vi "SIcamera_Manager- old.vi"() -> ()   [LabVIEW 2015]
uses:
  SI_Client_Subvis/Client Acquisition Mode Menu.ctl
  SI_Client_Subvis/Frame Mode 1.ctl
  SystemUtil/Command.ctl
  SI_Client_Subvis/CameraStates.ctl
  Log/LogItem.ctl
  GPS_Drivers/GPS_Driver_Global.vi
  TCS_Link/TCSLINK_global.vi
  Instance          36 24Saved   SIcamera_Manager .vi
  GUI/GSP_GUI_global.vi
  Apogee_Global.vi
panel:
  in  "CCD ROI Mode":u16(ring)=10 items=["Imaging, 1x1  "=0, "Imaging, 2x2"=1, "Imaging, 3x3"=2, "Spectroscopic, 1x1"=3, "Spectroscopic, 2x2"=4, "Spectroscopic, 3x3"=5, "MOS, 1x1"=11, "MOS, 2x2"=12, "MOS, 3x3"=13, "Slicer"=6, "Spectroscopic, ZZ Ceti"=14, "Slit Imaging/Alignment"=7, "MOS Imaging/Alignment"=10, "Set user-defined ROI..."=8, "Custom Mode"=9]
  in  "MOS":bool
  in  "Save As":u16(ring)=1 items=["U16 FITS", "I16 FITS", "I32 FITS", "SGL FITS", "U16 TIFF", "I16 TIFF", "I32 TIFF", "SGL TIFF"]
  in  "Port Readout":u16(ring)=2 items=["4-port", "Port A", "Port B", "Port C", "Port D"]
  in  "Lamp Cluster":T1
  out "Current File Name":string
  in  "Calculate Offset":bool
  in  "sy1":dbl
  in  "sx1":dbl
  in  "oy1":dbl
  in  "ox1":dbl
  in  "N/S Offset":dbl min=0.0 max=420.0 step=0.15 format="%03.2f"
  in  "N/S Offset Choice":u16(ring) items=["North", "South"]
  in  "E/W Offset Choice":u8(ring) items=["East", "West"]
  in  "E/W Offset":dbl min=0.0 max=420.0 step=0.15 format="%03.2f"
  in  "Offset Telescope":bool
  out "TCP/IP ID":refnum<k5>
  in  "Systems Status & Control":enum32{"Camera TCP/IP", "General"}(tab)
  in  "Reset TCP":bool
  in  "Get Camera Status":bool
  out "CCD Temp.":sgl
  out "Vacuum Pressure":sgl format="%#.4g"
  out "Connection Status":bool
  in  "Port":u16=2055
  in  "Server Address":string="Localhost"
  in  "Reset Wavelength Angles System":bool
  in  "Proposal #":string
  in  "Observer Name":string
  in  "Show Images?":bool
  out "CCD ROI":cluster{i32, i32, i32, i32, i32, i32}={0, 4096, 1, 0, 4096, 1}
  in  "CCD Readout Speed":u8(ring)=5 items=["50 kHz, ATTN 0", "50 kHz, ATTN 2", "50 kHz, ATTN 3", "100 kHz, ATTN 0", "100 kHz, ATTN 2", "100 kHz, ATTN 3", "200 kHz, ATTN 0", "200 kHz, ATTN 2", "400 kHz, ATTN 0"]
  out "Open Shutter During Image?":bool=TRUE
  out "Readout Time":dbl
  out "Image File Name":string="0001.image.fits"
  in  "Image #":i32=1 min=1 step=1 format="%04.0f"
  in  "Thumbnail Setting":enum16{"Check Entire CCD", "Check Star Focus"}(ring)
  in  "Take Thumbnail":bool
  out "Current Status":string
  in  "Save":bool
  in  "Frames":i32=1 min=1 step=1
  in  "Frame Mode":T2 items=["Single Frame Buffer", "Multiple Frame Buffer"]
  in  "Exp. Time (s)":dbl=1.0 min=0.5 step=1.0 format="%.1f"
  out "Packet\nError code":i32
  out "Function #":u16
  in  "# to Average":u32=2 caption="of"
  in  "RO Done":bool
  out "% Exposure":u16(slide) scale=0.0..100.0
  out "% Complete":u16(slide) caption="% Readout" scale=0.0..100.0
  out "Error out":errorcluster
  out "Acquiring":u32
  out "P Len":i32
  out "S Len":i32
  in  "Mode":u16(ring)=4 items=["Retrieve Image Buffer", "Acquire and transfer to client", "Acquire and hold in Server Image Buffer", "Acquire, transfer to client, and save to Server's disk", "Acquire, save to Server's disk, and hold in Server Image Buffer"]
  in  "Acq Mode":T3 caption="Acquisition Mode"
  in  "File Name Base":string="image"
  in  "SHUTDOWN":bool
  in  "Start Exposure":bool
  in  "Exposure Tab":enum32{"Object", "Flat", "Comp", "Dark", "Zero"}(tab)=enum."Zero"
  in  "# Exposures":i32=1 min=1 step=1
  in  "Object Comments:":string
  in  "Object Name:":string
  in  "Quartz Intensity":i8=70 caption="%" min=0 max=100 step=1
  in  "# Flat Exposures":i32=1 min=1 step=1
  in  "Flat Comments:":string
  in  "Flat Name:":string
  in  "# Comp Exposures":i32=1 min=1 step=1
  in  "Comp Comments:":string
  in  "Comp Name:":string
  out "Dark Name:":string="DARK"
  in  "Dark Comments:":string
  in  "# Dark Exposures":i32=1 min=1 step=1
  out "Zero Name:":string="ZERO"
  in  "Zero Comments:":string
  in  "# Zero Exposures":i32=1 min=1 step=1
  in  "Script":T4={"Exposure Time"=0.0, "#Exposures"=1, "Current Exposure"=2, "Last Exposure Start Time"=92278252, "Exposure type"=1, "Obs parameters"={"Object Name"="", "Telescope"="SOAR 4.1m", "Instrument"="Goodman Spectrograph", "Comment"=""}, "System Pos Info"={"Grating#"=0, "Slit#"=0, "Primary Filter#"=0, "Secondary Filter#"=0, "Coll Position"=1000, "Camera Focus"=-396, "Camera Angle"=12.21, "Grating Angle"=20.740599999999997, "Coll Temp"=0.0, "Cam Temp"=0.0, "Camera Target"=12.21, "Grating Target"=20.740599999999997}, "TCSInfo"={"Mount Az"=90.0001, "Mount El"=88.5355, "RA"="22:24:06.462", "DEC"="-30:13:35.702", "Hour Angle"="-00:04:55.6", "Airmass"=1.0, "Focus"=-1704.0, "Rotator Angle"=180.166, "Rotator Location"="", "Dome Shutter"="0.0071", "Dome Az"=319.9706, "Date"="2008-07-17", "UT Time"="19:06:13.7", "Sidereal Time"="22:24:06.462", "Position Angle"=360.0, "Seeing"=4.57, "OBSRA"="22:24:06.462", "OBSDEC"="22:24:06.462", "ADCSTAT"="22:24:06.462", "ADCPOS"="22:24:06.462"}, "Exposure Active?"=FALSE, "Component Names"={"Slit Name"="<NO MASK>", "F1_Name"="<NO FILTER>", "F2_Name"="<NO FILTER>", "Grating Name"="<NO GRATING>"}, "Other Info."={"CCD Read Noise"=3.99, "CCD Gain"=2.06, "OBSTYPE"="OBJECT", "OBSERVER"="", "Proposal #"="", "Equinox"=2000.0}, "Reduction Info."={"DISPAXIS"=1, "DETSIZE"="[1:4096,1:4096]", "CCDSUM"="1 1", "DETSEC"="[1:4096,1:4096]", "DATASEC"="[1:4096,1:4096]"}, "EnvironmentalInfo"={"Outside Temp"=0.0, "Wind Direction"=0.0, "Wind Speed"=0.0, "Pressure"=0.0, "Humidity"=0.0}} {"Other Info."."Equinox" format="%#.2f"; "Other Info."."CCD Gain" format="%#.2g"; "Other Info."."CCD Read Noise" format="%#.2g"; "Exposure type" items=["Dark", "Light"]}
  out "Camera Errors":errorcluster
  in  "CommandQ":string
  # "Save As"
  # "I16 FITS"
  # "Port Readout"
  # "Port B"
  # "x"
  # "y"
  # "Current Pixel Values:"
  # "\" to the"
  # "\" to the"
  # "Desired Pixel Values:"
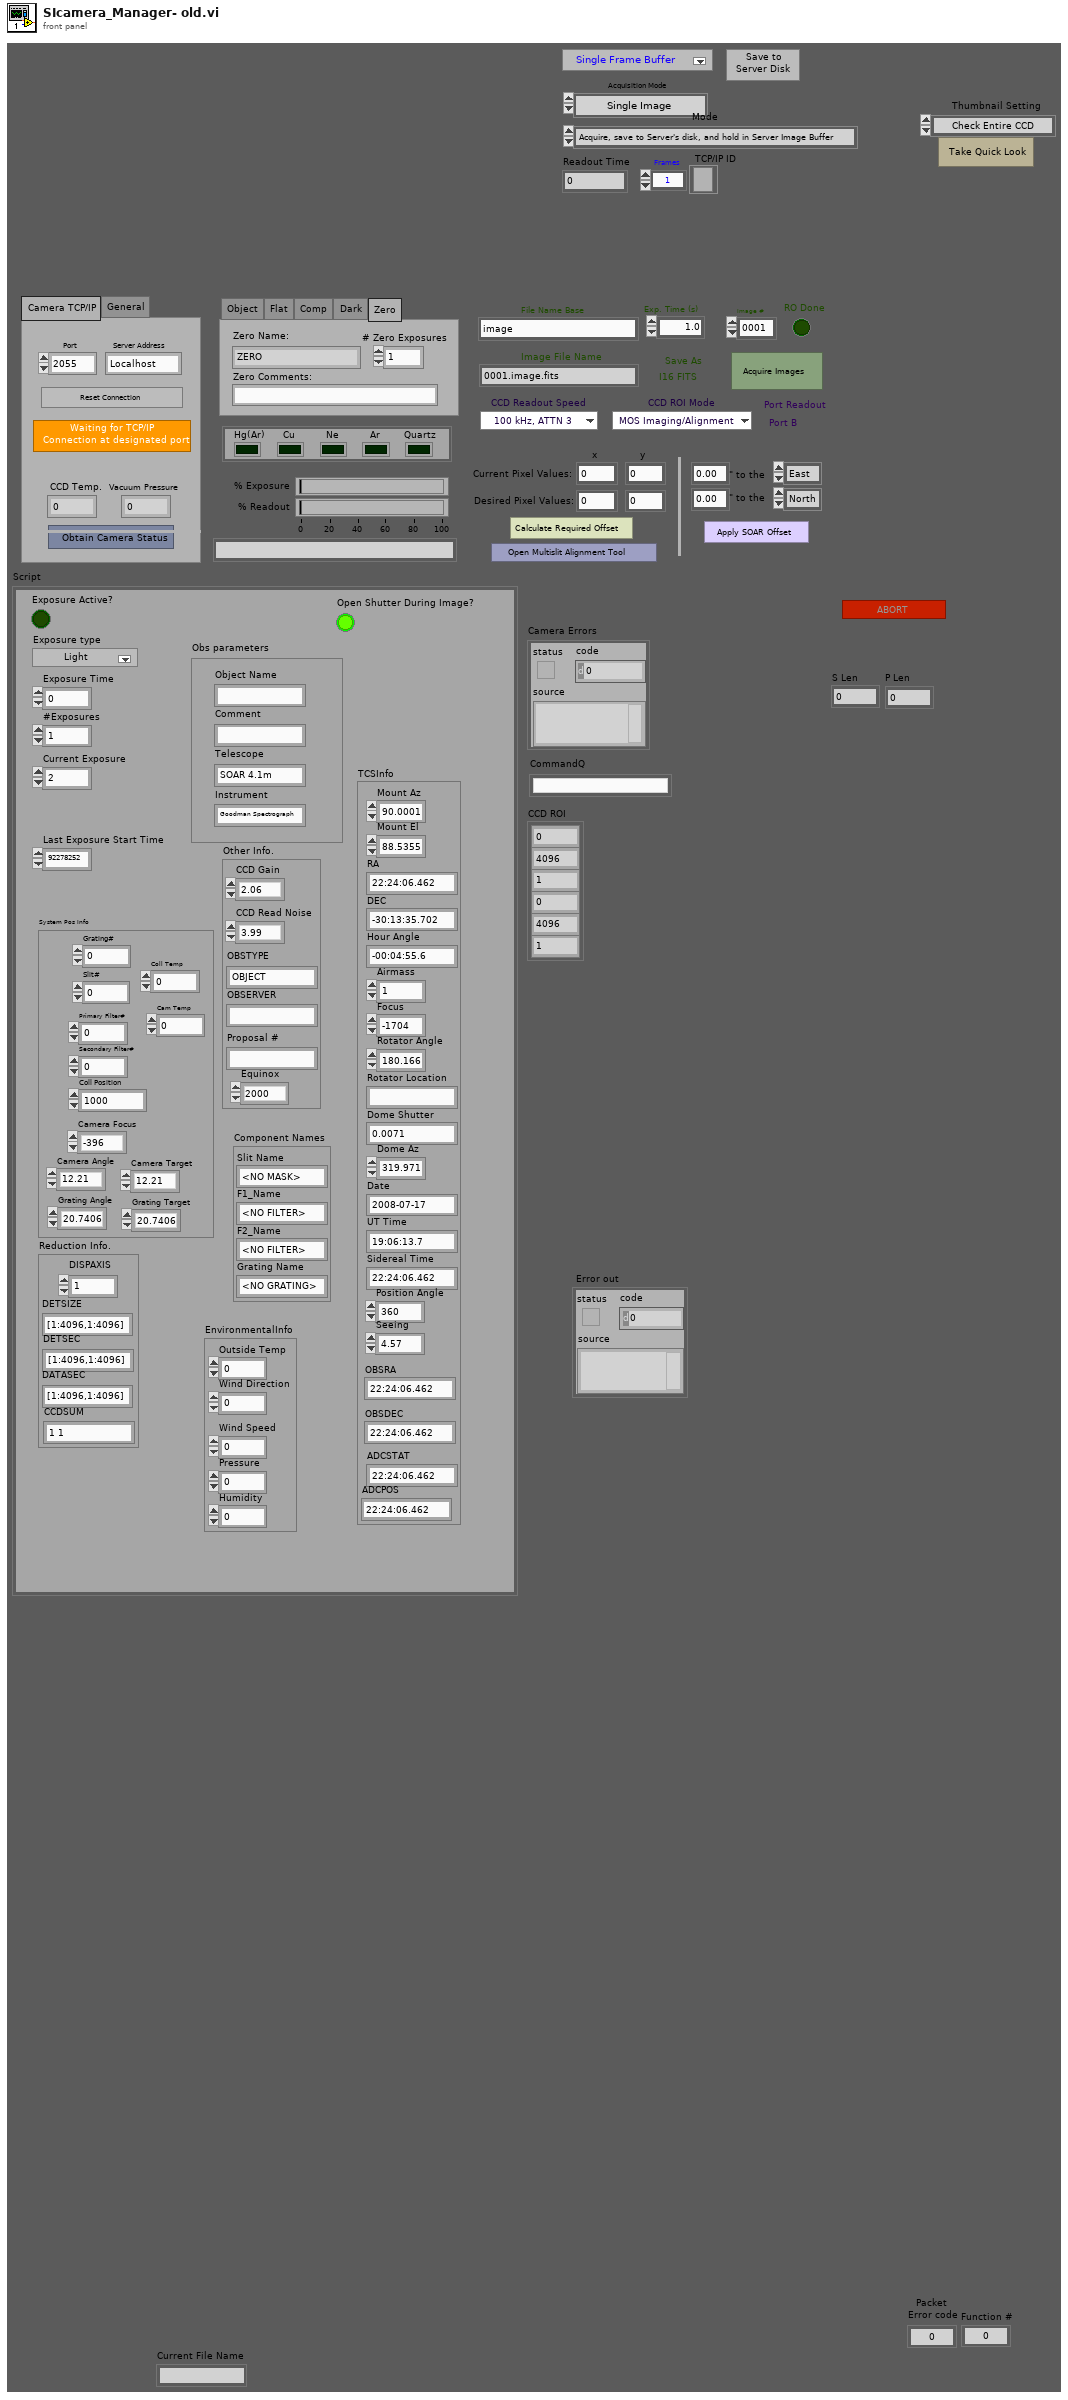
[diagram p1: front panel]
types:
  T1 = cluster{"Hg(Ar)":bool, "Cu":bool, "Ne":bool, "Ar":bool, "Quartz":bool}
  T2 = typedef "Frame Mode 1.ctl" = i32
  T3 = typedef "Client Acquisition Mode Menu.ctl" = enum16{"Single Image", "Average Images", "Multiple Frames"}
  T4 = cluster{"Exposure Time":dbl, "#Exposures":i32, "Current Exposure":i32, "Last Exposure Start Time":u32, "Exposure type":i16, "Obs parameters":cluster{"Object Name":string, "Telescope":string, "Instrument":string, "Comment":string}, "System Pos Info":cluster{"Grating#":i32, "Slit#":i32, "Primary Filter#":i32, "Secondary Filter#":i32, "Coll Position":i32, "Camera Focus":i32, "Camera Angle":dbl, "Grating Angle":dbl, "Coll Temp":dbl, "Cam Temp":dbl, "Camera Target":dbl, "Grating Target":dbl}, "TCSInfo":cluster{"Mount Az":dbl, "Mount El":dbl, "RA":string, "DEC":string, "Hour Angle":string, "Airmass":dbl, "Focus":dbl, "Rotator Angle":dbl, "Rotator Location":string, "Dome Shutter":string, "Dome Az":dbl, "Date":string, "UT Time":string, "Sidereal Time":string, "Position Angle":dbl, "Seeing":dbl, "OBSRA":string, "OBSDEC":string, "ADCSTAT":string, "ADCPOS":string}, "Exposure Active?":bool, "Component Names":cluster{"Slit Name":string, "F1_Name":string, "F2_Name":string, "Grating Name":string}, "Other Info.":cluster{"CCD Read Noise":dbl, "CCD Gain":dbl, "OBSTYPE":string, "OBSERVER":string, "Proposal #":string, "Equinox":dbl}, "Reduction Info.":cluster{"DISPAXIS":i8, "DETSIZE":string, "CCDSUM":string, "DETSEC":string, "DATASEC":string}, "EnvironmentalInfo":cluster{"Outside Temp":dbl, "Wind Direction":dbl, "Wind Speed":dbl, "Pressure":dbl, "Humidity":dbl}}
  T5 = typedef "Command.ctl" = cluster{"Command":string, "Parameter":string}
  T6 = cluster{"Object Name":string, "Telescope":string, "Instrument":string, "Comment":string}
  T7 = typedef "CameraStates.ctl" = enum16{"Ready", "Exposing", "Error"}
  T8 = enum16{"POL (0)", "CPL (1)", "HLT (2)", "STP (3)", "RST (4)", "RVN (5)", "RPB (6)", "CLP (8)", "SDL (9)", "RUN (10)", "WRI (11)", "RRG (12)", "SPR (13)", "LPR (14)", "VMI (15)", "SSP (17)", "SSE (18)", "RIS (20)", "RIO (21)", "IMW (25)", "END (128)", "MAV (134)", "MRV (135)", "JRE (137)", "WCL (138)", "WCW (139)", "DLY (140)", "WDL (141)", "GCL (142)", "GOP (143)", "ZTG (144)", "ZTP (145)", "TTP (146)", "CME (147)", "CTC (148)", "TQL (149)", "AHC (150)", "ERL (151)", "OLP (152)", "WRP (154)", "IDT (155)", "LRP (156)", "VMP (159)", "RAV (160)", "RRV (161)", "JMP (162)", "JOI (162)", "CIS (163)", "CKS (164)", "CLC (165)", "KMC (167)", "MCT (168)", "FLC (169)", "EEM (170)", "DDB (171)", "DEM (171)", "PAC (172)", "ADL (173)", "BRT (174)", "MAT (176)", "MRT (177)", "RAT (178)", "RRT (179)", "SSD (180)", "KMR (181)", "KED (182)", "KDD (183)", "DIR (184)", "PRO (185)", "SIF (186)", "EDL (187)", "CIO (188)", "MDS (189)", "MDC (190)", "MDT (191)", "SEE (192)", "ARI (193)", "WBS (194)", "SCF (195)", "RSM (196)", "RLM (197)", "RSN (198)", "RLN (199)", "PCL (201)", "PCI (201)", "PRT (202)", "PRI (202)", "WBE (204)", "SOB (205)", "COB (206)", "ACR (207)", "PLR (208)", "CAI (211)", "LVT (212)", "OVT (213)", "MTT (214)", "CLC (215)", "PIM (216)", "VIM (217)", "TIM (218)", "AHM (219)", "SSL (221)", "TRU (222)", "RSD (223)", "EMT (225)", "DMT (226)", "EMD (227)", "DMD (228)", "HSM (229)", "AHD (230)", "PCM (231)", "PCG (232)", "XRV (233)", "XAV (234)", "XRT (235)", "XAT (236)", "GOC (237)", "JNA (238)", "JOR (239)", "PMC (240)", "PMV (241)", "PMX (242)", "DLC (243)", "SLC (244)", "PCP (245)", "ATR (248)", "PMO (249)", "JAN (250)", "EDH (251)", "DIF (252)", "IMS (253)", "IMQ (254)"}
  T9 = typedef "LogItem.ctl" = cluster{"error in (no error)":errorcluster, "Source":string, "Comment ":string}
  T10 = enum16{"Launch", "Log", "Open", "Close", "Shutdown"}
  T11 = cluster{"Serial Origin":i32, "Serial Length":i32, "Serial Binning":i32, "Parallel Origin":i32, "Parallel Length":i32, "Parallel Binning":i32}
  T12 = cluster{"Mount Az":dbl, "Mount El":dbl, "RA":string, "DEC":string, "Hour Angle":string, "Airmass":dbl, "Focus":dbl, "Rotator Angle":dbl, "Rotator Location":string, "Dome Shutter":string, "Dome Az":dbl, "Date":string, "UT Time":string, "Sidereal Time":string, "Position Angle":dbl, "Seeing":dbl, "OBSRA":string, "OBSDEC":string, "Position ADC":string, "Position ADC 2":string}
  T13 = cluster{"Grating#":i32, "Slit#":i32, "Primary Filter#":i32, "Secondary Filter#":i32, "Coll Position":i32, "Camera Focus":i32, "Camera Angle":dbl, "Grating Angle":dbl, "Coll Temp":dbl, "CF Temp\n":dbl, "Camera Target":dbl, "Grating Target":dbl}
  T14 = cluster{"Slit Name":string, "F1_Name":string, "F2_Name":string, "Grating Name":string}
  T15 = cluster{"element":i32, "element":i32, "element":i32, "element":i32, "element":i32, "element":i32}
  T16 = cluster{"% Exp.":u16, "%Readout":u16, "Relative Pos.":u32}
  T17 = typedef "TCP-IP Image Packet.ctl" = cluster{"Image ID":u16, "Image Type":u16, "Serial Length":u16, "Parallel Length":u16, "# of Packets":u16, "Packet #":u16, "Offset":u32, "Image Bytes":u32, "Image Data $":string}
  T18 = cluster{"DISPAXIS":i8, "DETSIZE":string, "CCDSUM":string, "DETSEC":string, "DATASEC":string}
  T19 = cluster{"Grating#":i32, "Slit#":i32, "Primary Filter#":i32, "Secondary Filter#":i32, "Coll Position":i32, "Camera Focus":i32, "Camera Angle":dbl, "Grating Angle":dbl, "Coll Temp":dbl, "Cam Temp":dbl, "Camera Target":dbl, "Grating Target":dbl}
  T20 = cluster{"CCD Read Noise":dbl, "CCD Gain":dbl, "OBSTYPE":string, "OBSERVER":string, "Proposal #":string, "Equinox":dbl}
  T21 = cluster{"Exp. Time (s)":dbl, "CCD Read Noise":dbl, "CCD Gain":dbl, "OBSTYPE":string, "OBSERVER":string, "Proposal #":string, "Equinox":dbl}
  T22 = cluster{"Outside Temp":dbl, "Wind Direction":dbl, "Wind Speed":dbl, "Pressure":dbl, "Humidity":dbl}
  T23 = cluster{"Command":string, "Current File Name":string}
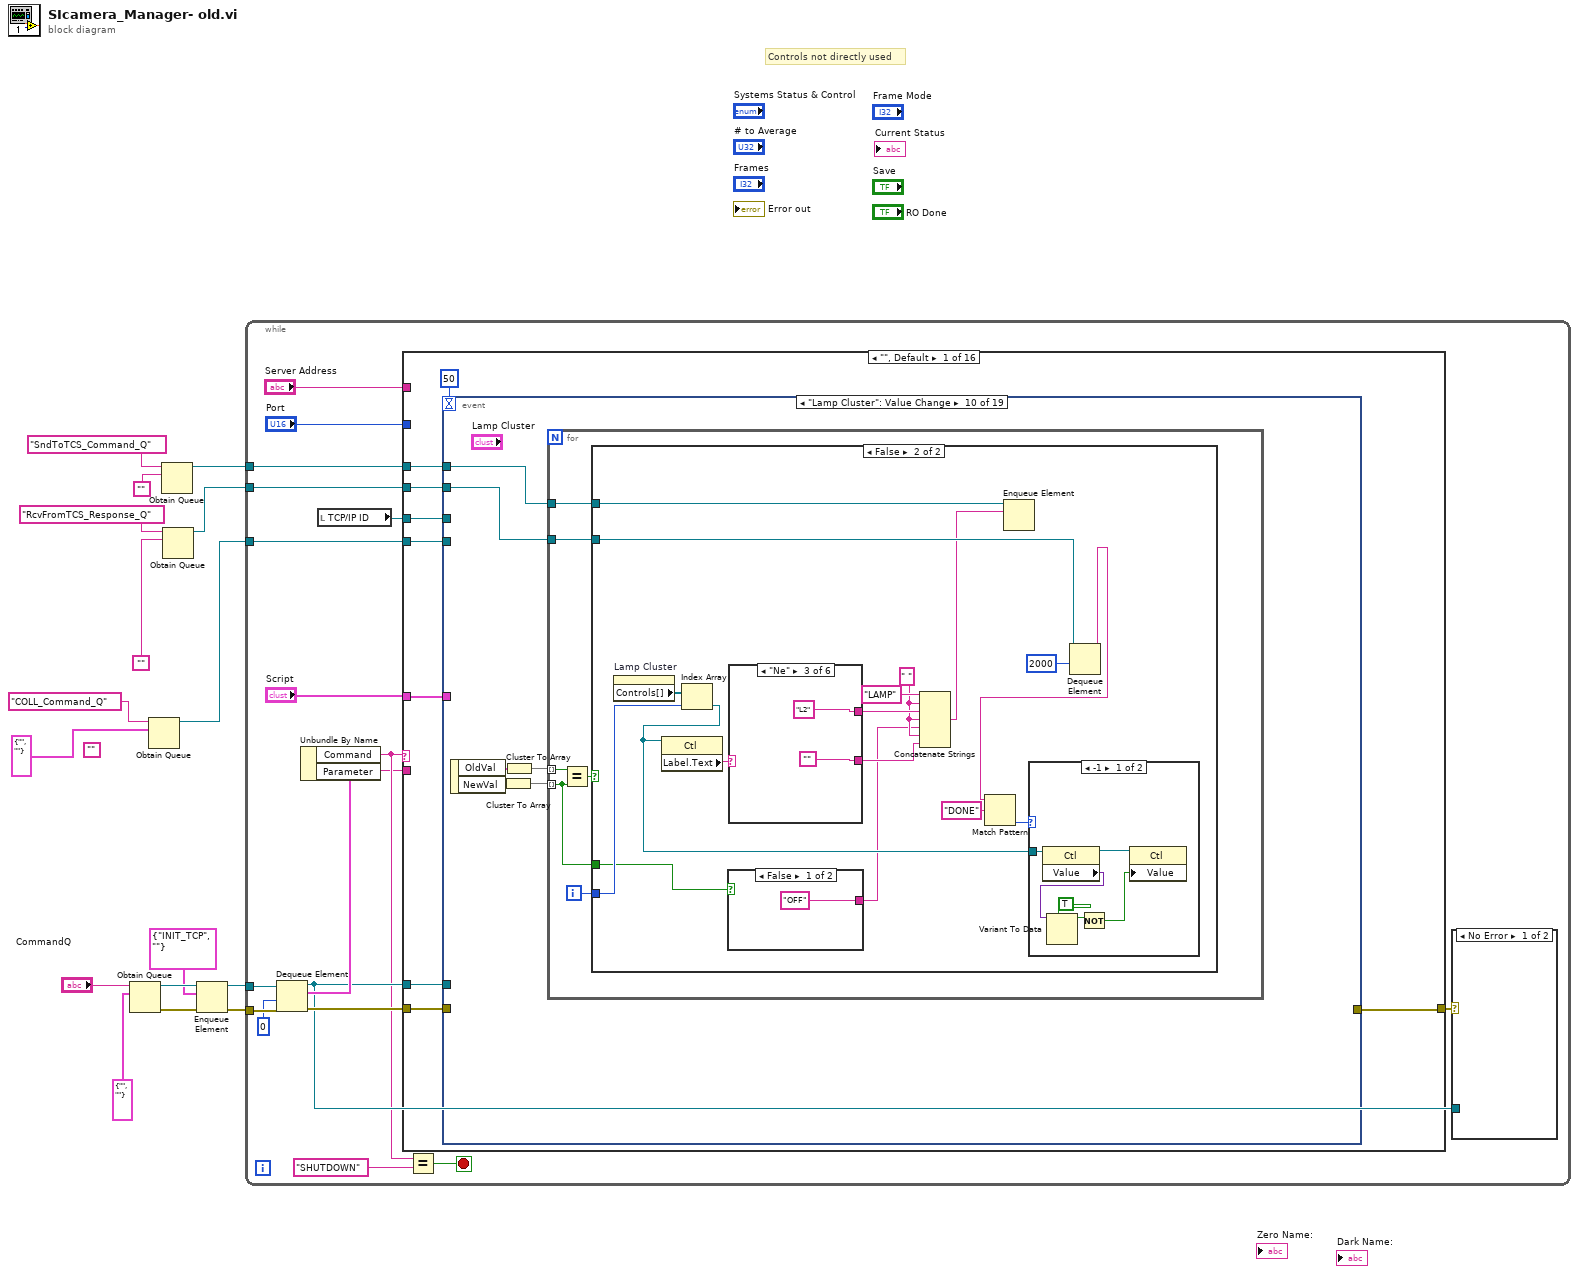
[diagram p0: block diagram]
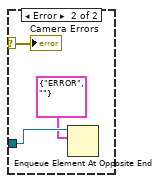
[diagram p2: hidden frame]
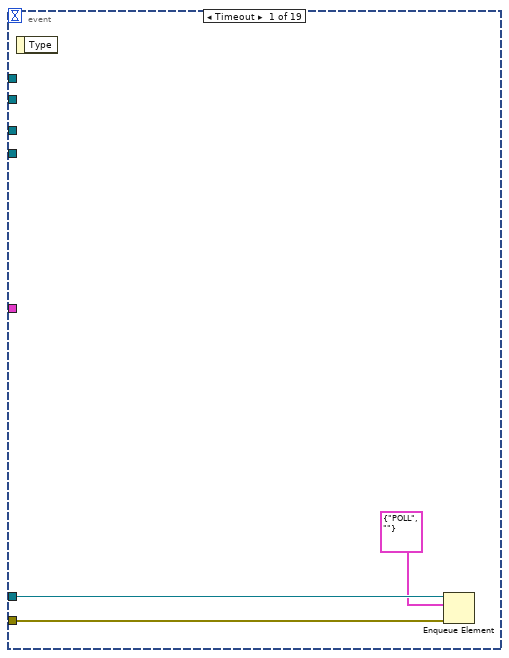
[diagram p3: hidden frame]
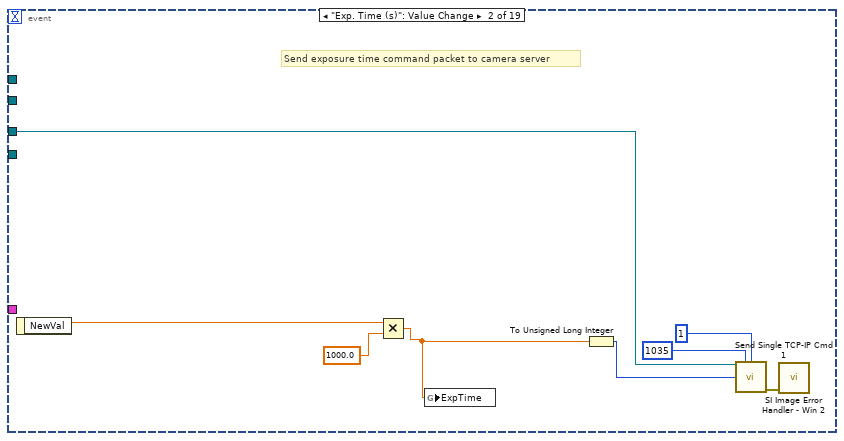
[diagram p4: hidden frame]
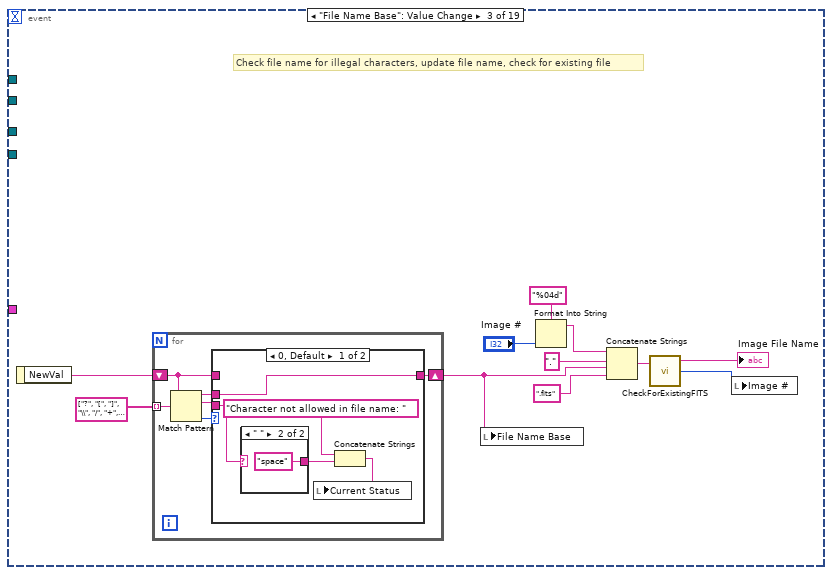
[diagram p5: hidden frame]
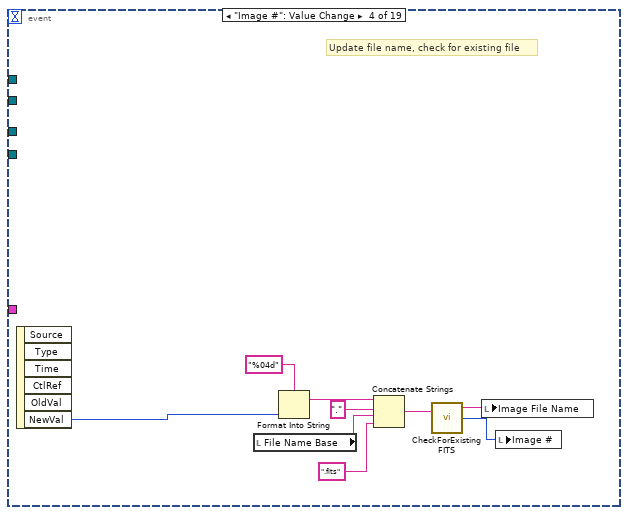
[diagram p8: hidden frame]
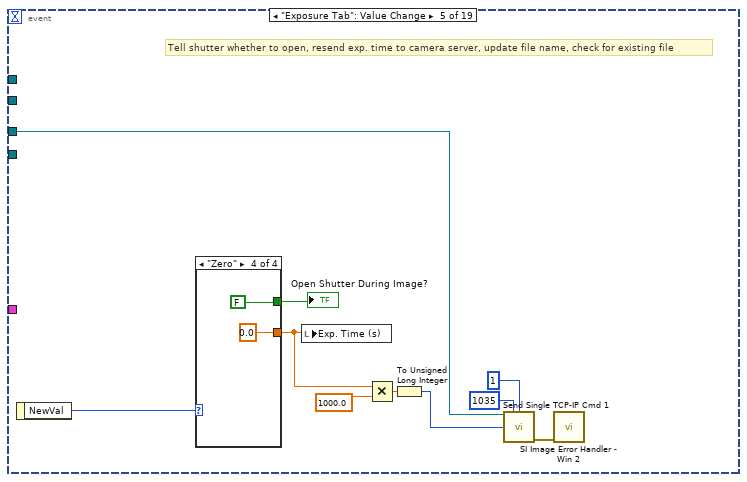
[diagram p9: hidden frame]
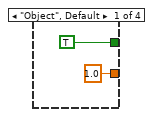
[diagram p10: hidden frame]
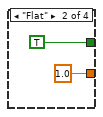
[diagram p11: hidden frame]
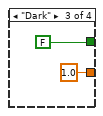
[diagram p12: hidden frame]
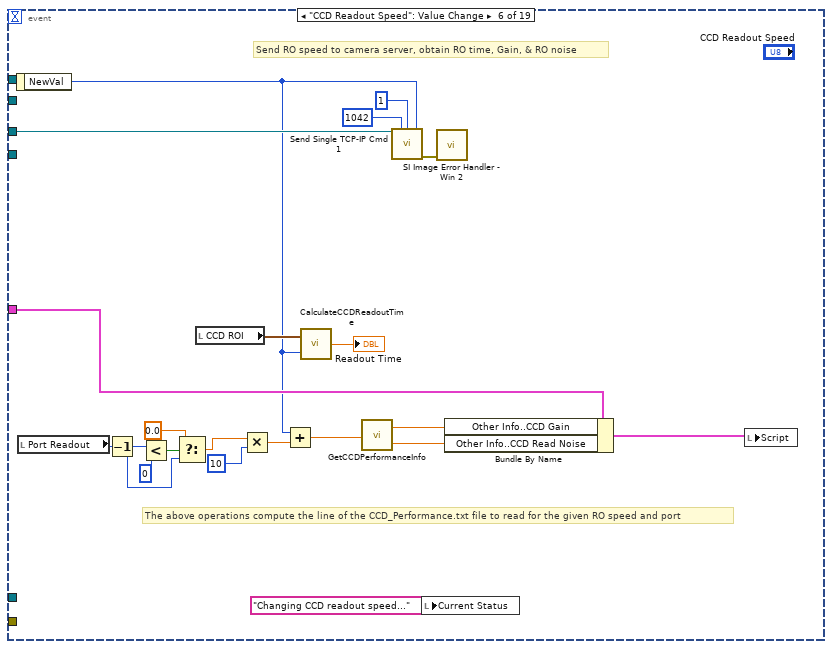
[diagram p13: hidden frame]
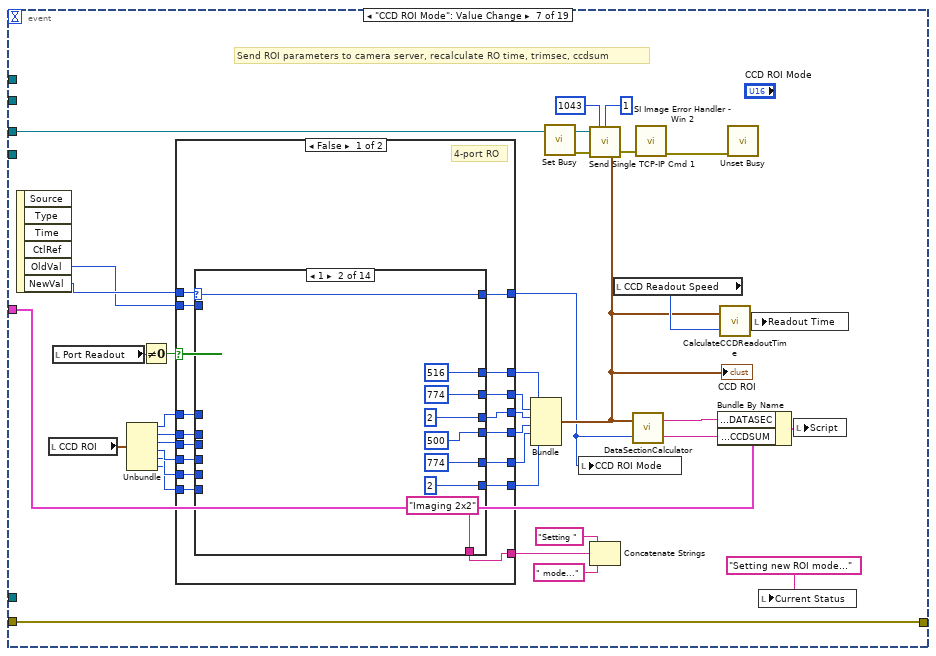
[diagram p14: hidden frame]
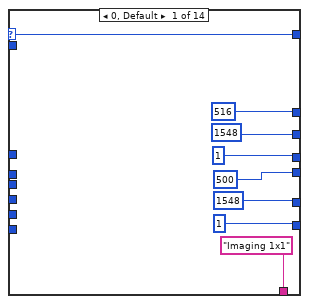
[diagram p15: hidden frame]
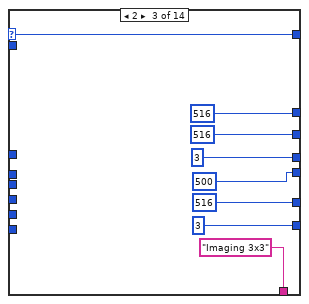
[diagram p16: hidden frame]
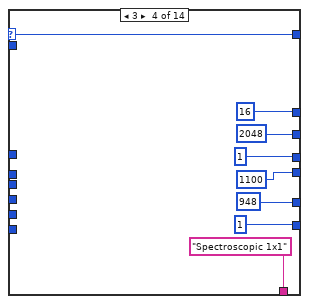
[diagram p17: hidden frame]
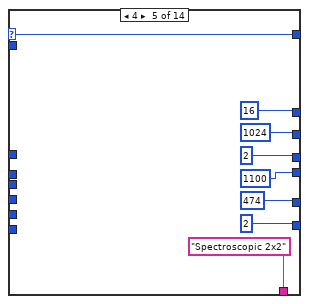
[diagram p18: hidden frame]
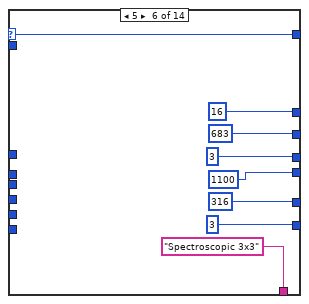
[diagram p19: hidden frame]
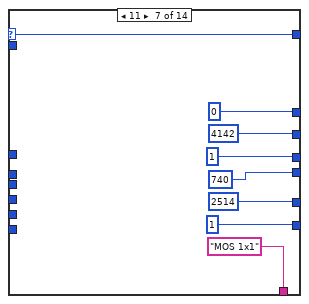
[diagram p20: hidden frame]
diagram:
  (unwired) ""
  # "Controls not directly used"
  n1 = Obtain Queue(name (unnamed)="CommandQ", element data type=T5 {"Command"="", "Parameter"=""} ("Command")) -> (queue out=w13:refnum<queue>, error out=w14:errorcluster)  [unwired: 3 in, 1 out]
  n2 = Obtain Queue(name (unnamed)="COLL_Command_Q", element data type=T5 {"Command"="", "Parameter"=""} ("Command")) -> (queue out=w3:refnum<queue>)  [unwired: 3 in, 2 out]
  n3 = Obtain Queue(name (unnamed)="SndToTCS_Command_Q", element data type="") -> (queue out=w7:refnum<queue>)  [unwired: 3 in, 2 out]
  n4 = Obtain Queue(name (unnamed)="RcvFromTCS_Response_Q", element data type="") -> (queue out=w4:refnum<queue>)  [unwired: 3 in, 2 out]
  n5 = Enqueue Element(queue=w13, element=T5 {"Command"="INIT_TCP", "Parameter"=""}, error in (no error)=w14) -> (queue out=w11:refnum<queue>, error out=w10:errorcluster)  [unwired: 1 in, 1 out]
  n6 = while {
    tunnel: w11 -> [w34]
    tunnel: w10 -> [w33]
    tunnel: w7 -> [w20]
    tunnel: w4 -> [w19]
    tunnel: w3 -> [w17]
    stop <- w24 stop-if-true
    n7 = Dequeue Element(queue=w34, timeout in ms (-1)=0, error in (no error)=w33) -> (queue out=w26:refnum<queue>, element=w31:T5, error out=w29:errorcluster)  [unwired: 1 out]
    n8 = Unbundle By Name(w31) -> ("Command"=w22:string, "Parameter"=w18:string)
    n9 = local read "TCP/IP ID"() -> (w21:refnum<k5>)
    n10 = case shown="\"\", Default" w22 {
      tunnel: w26 -> [w46 _ w764 _ w814 w902 _ _ w1168 _ _ _ _ _ w1312 w1351]
      tunnel: w29 -> [w45 w752 w767 w800 w812 w918 w1135 w1147 w1162 w1225 w1236 w1246 w1259 w1310 _ w1350]
      tunnel: "Port" -> [_ _ w769 _ _ _ _ _ _ _ _ _ _ _ _ _]
      tunnel: "Server Address" -> [_ _ w768 _ _ _ _ _ _ _ _ _ _ _ _ _]
      tunnel: [w43 w752 errorcluster {"status"=FALSE, "code"=0, "source"=""} ("error out") w781 w813 w918 w1105 w1147 w1167 w1224 w1236 w1246 w1254 w1310 errorcluster {"status"=FALSE, "code"=0, "source"=""} ("error out") w1347] -> w25
      tunnel: "Script" -> [w44 _ _ _ w815 w904 w1138 _ w1155 _ _ _ _ _ _ _]
      tunnel: w21 -> [w41 _ _ w804 w811 w903 _ _ w1159 _ _ _ w1255 _ _ w1344]
      tunnel: w20 -> [w40 _ _ _ _ _ _ _ _ _ _ _ _ _ _ w1343]
      tunnel: w19 -> [w39 _ _ _ _ _ _ _ _ _ _ _ _ _ _ w1342]
      tunnel: w18 -> [_ w755 _ _ _ _ _ _ _ _ _ _ _ _ _ _]
      tunnel: w17 -> [w38 _ _ _ _ _ _ w1141 _ _ _ _ _ w1308 _ _]
      frame "", Default {
        n11 = event shown="[9] \"Lamp Cluster\": Value Change" {
          selector: _ -> [_ _ _ _ _ _ _ _ _ _ _ _ _ _ _ _ _ _ _]
          dyn-events: _ -> [_ _ _ _ _ _ _ _ _ _ _ _ _ _ _ _ _ _ _]
          timeout: 50 -> [_ _ _ _ _ _ _ _ _ _ _ _ _ _ _ _ _ _ _]
          tunnel: w46 -> [w49 _ _ _ _ _ _ _ _ _ _ _ _ _ _ _ _ w739 w744]
          tunnel: w45 -> [w48 _ _ _ _ _ w159 _ _ _ w571 w590 _ _ _ _ _ w738 w743]
          tunnel: w44 -> [_ _ _ _ _ w123 w136 w473 _ _ _ w591 _ w658 _ _ _ _ _]
          tunnel: [_ _ _ _ _ _ w159 _ _ _ w570 w590 _ _ _ _ _ w734 w742] -> w43
          tunnel: w41 -> [_ w52 _ _ w94 w127 w144 w482 _ _ _ _ _ w659 _ _ _ w740 _]
          tunnel: w40 -> [_ _ _ _ _ _ _ _ _ w516 _ _ _ _ _ _ w713 _ _]
          tunnel: w39 -> [_ _ _ _ _ _ _ _ _ w515 _ _ _ _ _ _ w712 _ _]
          tunnel: w38 -> [_ _ _ _ _ _ _ _ _ _ _ _ _ _ _ _ _ _ _]
          event Timeout {
            n12 = event-data() -> ()  [unwired: 1 in, 1 out]
            n13 = Enqueue Element(queue=w49, element=T5 {"Command"="POLL", "Parameter"=""}, error in (no error)=w48) -> ()  [unwired: 1 in, 3 out]
          }
          event "Exp. Time (s)": Value Change {
            # "Send exposure time command packet to camera server"
            n14 = event-data() -> ("NewVal"=w50:dbl)  [unwired: 1 in]
            n15 = Multiply(x=w50, y=1000.0) -> (x*y=w51:dbl)
            n16 = global write "GPS_Driver_Global.vi" "ExpTime"(w51) -> ()
            n17 = To Unsigned Long Integer(number=w51) -> (unsigned 32bit integer=w57:u32)
            n18 = call "Send Single TCP-IP Cmd 1.vi"("TCP/IP ID"=w52, "Function #"=u16 1035, "Camera ID"=u8 1, "Exposure Time (ms)"=w57) -> ("Error Out"=w55:errorcluster)  [unwired: 8 in, 3 out]
            n19 = call "SI Image Error Handler - Win 2.vi"("error in (no error)"=w55) -> ()  [unwired: 4 in, 1 out]
          }
          event "File Name Base": Value Change {
            # "Check file name for illegal characters, update file name, check for existing file"
            n20 = event-data() -> ("NewVal"=w59:string)  [unwired: 1 in]
            n21 = for {
              tunnel: string[] ["?", "[", "]", "\\", "/", "=", "+", "<", ">", ":", ";", "\"", ",", " ", "*"] -> [w74] mode=indexing
              shift-right: [w70] -> w58
              shift-left: w59 -> [w71]
              n22 = Match Pattern(string=w71, regular expression=w74) -> (before substring=w72:string, match substring=w69:string, offset past match=w73:i32)  [unwired: 1 in, 1 out]
              n23 = case shown="0, Default" w73 {
                tunnel: w72 -> [w79 _]
                tunnel: w71 -> [_ w82]
                tunnel: [w79 w82] -> w70
                tunnel: w69 -> [w77 _]
                frame 0, Default {
                  n24 = case shown="\" \"" w77 {
                    selector: w77 -> [w80 _]
                    tunnel: [w80 "space"] -> w76
                    frame Default {
                    }
                    frame " " {
                    }
                  }
                  n25 = Concatenate Strings("Character not allowed in file name: " ("string"), w76) -> (w75:string)
                  n26 = local write "Current Status"(w75) -> ()
                }
                frame -1 {
                }
              }
            }
            n27 = local write "File Name Base"(w58) -> ()
            n28 = Format Into String(format string="%04d", "Image #") -> (resulting string=w66:string)  [unwired: 2 in, 1 out]
            n29 = Concatenate Strings(w66, "." ("string"), w58, ".fits" ("string")) -> (w62:string)
            n30 = call "CheckForExistingFITS.vi"("Filename"=w62) -> ("New Filename"=→"Image File Name":string, "New Exposure #"=w63:i32)  [unwired: 1 in, 1 out]
            n31 = local write "Image #"(w63) -> ()
          }
          event "Image #": Value Change {
            # "Update file name, check for existing file"
            n32 = event-data() -> ("NewVal"=w90:i32)  [unwired: 1 in, 5 out]
            n33 = local read "File Name Base"() -> (w87:string)
            n34 = Format Into String(format string="%04d", w90) -> (resulting string=w89:string)  [unwired: 2 in, 1 out]
            n35 = Concatenate Strings(w89, "." ("string"), w87, ".fits" ("string")) -> (w85:string)
            n36 = call "CheckForExistingFITS.vi"("Filename"=w85) -> ("New Filename"=w84:string, "New Exposure #"=w83:i32)  [unwired: 1 in, 1 out]
            n37 = local write "Image File Name"(w84) -> ()
            n38 = local write "Image #"(w83) -> ()
          }
          event "Exposure Tab": Value Change {
            # "Tell shutter whether to open, resend exp. time to camera server, update file name, check for existing file"
            n39 = event-data() -> ("NewVal"=w101:enum32{"Object", "Flat", "Comp", "Dark", "Zero"})  [unwired: 1 in]
            n40 = case shown="\"Zero\"" w101 {
              tunnel: [1.0 ("Exposure Time") 1.0 ("Exposure Time") 1.0 ("Exposure Time") 0.0 ("Exposure Time")] -> w93
              tunnel: [TRUE ("Open Shutter During Image?") TRUE ("Open Shutter During Image?") FALSE ("Open Shutter During Image?") FALSE ("Open Shutter During Image?")] -> w92
              frame "Object", Default {
              }
              frame "Flat" {
              }
              frame "Dark" {
              }
              frame "Zero" {
              }
            }
            "Open Shutter During Image?" <- w92
            n41 = local write "Exp. Time (s)"(w93) -> ()
            n42 = Multiply(x=w93, y=1000.0) -> (x*y=w99:dbl)
            n43 = To Unsigned Long Integer(number=w99) -> (unsigned 32bit integer=w100:u32)
            n44 = call "Send Single TCP-IP Cmd 1.vi"("TCP/IP ID"=w94, "Function #"=u16 1035, "Camera ID"=u8 1, "Exposure Time (ms)"=w100) -> ("Error Out"=w97:errorcluster)  [unwired: 8 in, 3 out]
            n45 = call "SI Image Error Handler - Win 2.vi"("error in (no error)"=w97) -> ()  [unwired: 4 in, 1 out]
          }
          event "CCD Readout Speed": Value Change {
            # "The above operations compute the line of the CCD_Performance.txt file to read for the given RO speed and port"
            # "Send RO speed to camera server, obtain RO time, Gain, & RO noise"
            n46 = event-data() -> ("NewVal"=w116:u8)  [unwired: 1 in]
            n47 = local read "Port Readout"() -> (w112:u16)
            n48 = Decrement(x=w112) -> (x-1=w110:u16)
            n49 = Less?(x=w110, y=u16 0) -> (x < y?=w114:bool)
            n50 = Select(t=0.0, s=w114, f=w110) -> (s? t:f=w111:dbl)
            n51 = local read "CCD ROI"() -> (w126:cluster{i32, i32, i32, i32, i32, i32})
            n52 = Multiply(x=w111, y=u16 10) -> (x*y=w117:dbl)
            n53 = Add(x=w116, y=w117) -> (x+y=w118:dbl)
            n54 = call "CalculateCCDReadoutTime.vi"("Readout Speed"=w116, "CCD ROI"=w126) -> ("Readout Time"=→"Readout Time":dbl)
            n55 = call "GetCCDPerformanceInfo.vi"("RO Speed Mode"=w118) -> ("Gain"=w122:dbl, "Read Noise"=w121:dbl)
            n56 = call "Send Single TCP-IP Cmd 1.vi"("TCP/IP ID"=w127, "Function #"=u16 1042, "Camera ID"=u8 1, "Acq. Mode/Type/Frame Mode/RO Mode #"=w116) -> ("Error Out"=w130:errorcluster)  [unwired: 8 in, 3 out]
            n57 = local write "Current Status"("Changing CCD readout speed..." ("Current Status")) -> ()
            n58 = call "SI Image Error Handler - Win 2.vi"("error in (no error)"=w130) -> ()  [unwired: 4 in, 1 out]
            n59 = Bundle By Name(cluster=w123, "Other Info..CCD Gain"=w122, "Other Info..CCD Read Noise"=w121) -> (w120:T4)
            n60 = local write "Script"(w120) -> ()
          }
          event "CCD ROI Mode": Value Change {
            # "Send ROI parameters to camera server, recalculate RO time, trimsec, ccdsum"
            n61 = event-data() -> ("OldVal"=w131:u16, "NewVal"=w132:u16)  [unwired: 1 in, 4 out]
            n62 = local read "CCD ROI"() -> (w151:cluster{i32, i32, i32, i32, i32, i32})
            n63 = local read "Port Readout"() -> (w156:u16)
            n64 = Unbundle(w151) -> (w150:i32, w149:i32, w148:i32, w147:i32, w146:i32, w145:i32)
            n65 = Not Equal To 0?(x=w156) -> (x != 0?=w155:bool)
            n66 = case shown="False" w155 {
              tunnel: w132 -> [w168 w324]
              tunnel: [w182 w323] -> w164
              tunnel: [w181 w322] -> w163
              tunnel: [w180 w321] -> w139
              tunnel: [w179 w320] -> w162
              tunnel: [w178 w319] -> w161
              tunnel: [w177 w318] -> w160
              tunnel: [w176 w317] -> w141
              tunnel: w150 -> [w175 w316]
              tunnel: w149 -> [w174 w315]
              tunnel: w148 -> [w173 w314]
              tunnel: w147 -> [w172 w313]
              tunnel: w146 -> [w171 w312]
              tunnel: w145 -> [w170 w311]
              tunnel: w131 -> [w169 w310]
              tunnel: [w167 w309] -> w137
              frame False {
                # "4-port RO"
                n67 = case shown="1" w168 {
                  selector: w168 -> [w183 w191 w199 w207 w215 w223 w231 w239 w247 w255 w270 w271 w286 _]
                  tunnel: [516 516 516 16 16 16 0 0 0 0 0 1850 1366 w301] -> w182
                  tunnel: [1548 774 516 2048 1024 683 4142 2071 1381 2071 2071 200 1370 w300] -> w181
                  tunnel: [1 2 3 1 2 3 1 2 3 2 2 1 1 w299] -> w180
                  tunnel: [500 500 500 1100 1100 1100 740 740 740 1800 980 1100 790 w298] -> w179
                  tunnel: [1548 774 516 948 474 316 2514 1257 838 200 1008 948 2370 w297] -> w178
                  tunnel: [1 2 3 1 2 3 1 2 3 2 2 1 1 w296] -> w177
                  tunnel: ["Imaging 1x1" ("Current Status") "Imaging 2x2" ("Current Status") "Imaging 3x3" ("Current Status") "Spectroscopic 1x1" ("Current Status") "Spectroscopic 2x2" ("Current Status") "Spectroscopic 3x3" ("Current Status") "MOS 1x1" ("Current Status") "MOS 2x2" ("Current Status") "MOS 3x3" ("Current Status") "Spectroscopic ZZ Ceti" ("Current Status") "Slicer" ("Current Status") "Slit Imaging/Alignment" ("Current Status") "MOS Imaging/Alignment" ("Current Status") "user-defined" ("Current Status")] -> w176
                  tunnel: w175 -> [_ _ _ _ _ _ _ _ _ _ _ _ _ w294]
                  tunnel: w174 -> [_ _ _ _ _ _ _ _ _ _ _ _ _ w293]
                  tunnel: w173 -> [_ _ _ _ _ _ _ _ _ _ _ _ _ w292]
                  tunnel: w172 -> [_ _ _ _ _ _ _ _ _ _ _ _ _ w291]
                  tunnel: w171 -> [_ _ _ _ _ _ _ _ _ _ _ _ _ w290]
                  tunnel: w170 -> [_ _ _ _ _ _ _ _ _ _ _ _ _ w289]
                  tunnel: w169 -> [_ _ _ _ _ _ _ _ _ _ _ _ _ w288]
                  tunnel: [w183 w191 w199 w207 w215 w223 w231 w239 w247 w255 w270 w271 w286 w287] -> w167
                  frame 0, Default {
                  }
                  frame 1 {
                  }
                  frame 2 {
                  }
                  frame 3 {
                  }
                  frame 4 {
                  }
                  frame 5 {
                  }
                  frame 11 {
                  }
                  frame 12 {
                  }
                  frame 13 {
                  }
                  frame 14 {
                  }
                  frame 6 {
                  }
                  frame 7 {
                  }
                  frame 10 {
                  }
                  frame 8, 9 {
                    n68 = call "GetCCDParameters.vi"("Serial Origin"=w294, "Parallel Origin"=w291, "Serial Length"=w293, "Parallel Length"=w290, "Serial Binning"=w292, "Parallel Binning"=w289) -> ("Cancelled?"=w303:bool, "CCD Format Parameters"=w304:T11)  [unwired: 10 in, 2 out]
                    n69 = case shown="False" w303 {
                      tunnel: w304 -> [w306 _]
                      tunnel: [w306 w308] -> w302
                      tunnel: w288 -> [_ w307]
                      tunnel: [u8 8 ("Camera ID") w307] -> w287
                      frame False {
                      }
                      frame True {
                        n70 = local read "CCD ROI"() -> (w308:cluster{i32, i32, i32, i32, i32, i32})
                      }
                    }
                    n71 = Unbundle(w302) -> ("Serial Origin"=w301:i32, "Serial Length"=w300:i32, "Serial Binning"=w299:i32, "Parallel Origin"=w298:i32, "Parallel Length"=w297:i32, "Parallel Binning"=w296:i32)
                  }
                }
              }
              frame True {
                # "1-port RO"
                n72 = case shown="2" w324 {
                  selector: w324 -> [w325 w333 w341 w349 w357 w365 w373 w381 w389 w397 w412 w413 w421 _]
                  tunnel: [516 516 516 0 0 0 0 0 0 0 0 1850 1366 w443] -> w323
                  tunnel: [3096 1548 1032 4142 2071 1381 4142 2071 1381 2071 2071 400 1370 w442] -> w322
                  tunnel: [1 2 3 1 2 3 1 2 3 2 2 1 1 w441] -> w321
                  tunnel: [500 500 500 1100 1100 1100 740 740 740 1800 980 1100 790 w440] -> w320
                  tunnel: [3096 1548 1032 1896 948 632 2514 1257 838 200 1048 1896 2370 w439] -> w319
                  tunnel: [1 2 3 1 2 3 1 2 3 2 2 1 1 w438] -> w318
                  tunnel: ["Imaging 1x1" ("Current Status") "Imaging 2x2" ("Current Status") "Imaging 3x3" ("Current Status") "Spectroscopic 1x1" ("Current Status") "Spectroscopic 2x2" ("Current Status") "Spectroscopic 3x3" ("Current Status") "MOS 1x1" ("Current Status") "MOS 2x2" ("Current Status") "MOS 3x3" ("Current Status") "Spectroscopic ZZ Ceti" ("Current Status") "Slicer" ("Current Status") "Slit Imaging/Alignment" ("Current Status") "MOS Imaging/Alignment" ("Current Status") "user-defined" ("Current Status")] -> w317
                  tunnel: w316 -> [_ _ _ _ _ _ _ _ _ _ _ _ _ w436]
                  tunnel: w315 -> [_ _ _ _ _ _ _ _ _ _ _ _ _ w435]
                  tunnel: w314 -> [_ _ _ _ _ _ _ _ _ _ _ _ _ w434]
                  tunnel: w313 -> [_ _ _ _ _ _ _ _ _ _ _ _ _ w433]
                  tunnel: w312 -> [_ _ _ _ _ _ _ _ _ _ _ _ _ w432]
                  tunnel: w311 -> [_ _ _ _ _ _ _ _ _ _ _ _ _ w431]
                  tunnel: w310 -> [_ _ _ _ _ _ _ _ _ _ _ _ _ w430]
                  tunnel: [w325 w333 w341 w349 w357 w365 w373 w381 w389 w397 w412 w413 w421 w429] -> w309
                  frame 0, Default {
                  }
                  frame 1 {
                  }
                  frame 2 {
                  }
                  frame 3 {
                  }
                  frame 4 {
                  }
                  frame 5 {
                  }
                  frame 11 {
                  }
                  frame 12 {
                  }
                  frame 13 {
                  }
                  frame 14 {
                  }
                  frame 6 {
                  }
                  frame 7 {
                  }
                  frame 10 {
                  }
                  frame 8, 9 {
                    n73 = call "GetCCDParameters.vi"("Serial Origin"=w436, "Parallel Origin"=w433, "Serial Length"=w435, "Parallel Length"=w432, "Serial Binning"=w434, "Parallel Binning"=w431) -> ("Cancelled?"=w445:bool, "CCD Format Parameters"=w444:T11)  [unwired: 10 in, 2 out]
                    n74 = case shown="False" w445 {
                      tunnel: w444 -> [w453 _]
                      tunnel: [w452 w460] -> w443
                      tunnel: [w451 w459] -> w442
                      tunnel: [w450 w458] -> w441
                      tunnel: [w449 w457] -> w440
                      tunnel: [w448 w456] -> w439
                      tunnel: [w447 w455] -> w438
                      tunnel: w430 -> [_ w454]
                      tunnel: [u8 8 ("Camera ID") w454] -> w429
                      frame False {
                        n75 = Unbundle(w453) -> ("Serial Origin"=w452:i32, "Serial Length"=w451:i32, "Serial Binning"=w450:i32, "Parallel Origin"=w449:i32, "Parallel Length"=w448:i32, "Parallel Binning"=w447:i32)
                      }
                      frame True {
                        n76 = local read "CCD ROI"() -> (w461:cluster{i32, i32, i32, i32, i32, i32})
                        n77 = Unbundle(w461) -> (w460:i32, w459:i32, w458:i32, w457:i32, w456:i32, w455:i32)
                      }
                    }
                  }
                }
              }
            }
            n78 = Bundle("Serial Origin"=w164, "Serial Length"=w163, "Serial Binning"=w139, "Parallel Origin"=w162, "Parallel Length"=w161, "Parallel Binning"=w160) -> (w138:T11)  [unwired: 1 in]
            "CCD ROI" <- w138
            n79 = call <vilib>:"Set Busy.vi"() -> ("error out"=w143:errorcluster)  [unwired: 10 in, 1 out]
            n80 = local write "CCD ROI Mode"(w137) -> ()
            n81 = call "Send Single TCP-IP Cmd 1.vi"("TCP/IP ID"=w144, "Function #"=u16 1043, "Camera ID"=u8 1, "Error In"=w143, "CCD Format Parameters"=w138) -> ("Error Out"=w158:errorcluster)  [unwired: 7 in, 3 out]
            n82 = Concatenate Strings("Setting " ("string"), w141, " mode..." ("Current Status")) -> ()  [unwired: 1 out]
            n83 = local read "CCD Readout Speed"() -> (w153:u8)
            n84 = call "DataSectionCalculator.vi"("Standard Mode #"=w137, "CCD ROI"=w138) -> ("CCDSUM"=w134:string, "TRIMSEC"=w135:string)
            n85 = call "SI Image Error Handler - Win 2.vi"("error in (no error)"=w158) -> ("error out"=w142:errorcluster)  [unwired: 4 in]
            n86 = Bundle By Name(cluster=w136, "Reduction Info..DATASEC"=w135, "Reduction Info..CCDSUM"=w134) -> (w133:T4)
            n87 = call "CalculateCCDReadoutTime.vi"("Readout Speed"=w153, "CCD ROI"=w138) -> ("Readout Time"=w154:dbl)
            n88 = call <vilib>:"Unset Busy.vi"("error in (no error)"=w142) -> ()  [unwired: 10 in, 1 out]
            n89 = local write "Readout Time"(w154) -> ()
            n90 = local write "Current Status"("Setting new ROI mode..." ("Current Status")) -> ()
            n91 = local write "Script"(w133) -> ()
          }
          event "Port Readout": Value Change {
            w479 = u8 5 items=["50 kHz, ATTN 0", "50 kHz, ATTN 2", "50 kHz, ATTN 3", "100 kHz, ATTN 0", "100 kHz, ATTN 2", "100 kHz, ATTN 3", "200 kHz, ATTN 0", "200 kHz, ATTN 2", "400 kHz, ATTN 0"] ("CCD Readout Speed")
            # "Send camera server mode number to read from .set file to set correct port readout choice, get GAIN & RO noise"
            # "Can remove this once I take care of all of the RO speed possibilties for port modes in *.set file"
            # "Add 9 because there are nine previous modes before getting to Port-changing modes in .set file"
            n92 = event-data() -> ("NewVal"=w463:u16)  [unwired: 1 in, 1 out]
            n93 = Decrement(x=w463) -> (x-1=w462:u16)
            n94 = Less?(x=w462, y=u16 0) -> (x < y?=w468:bool)
            n95 = Select(t=0.0, s=w468, f=w462) -> (s? t:f=w466:dbl)
            n96 = Multiply(x=w466, y=u16 10) -> (x*y=w470:dbl)
            n97 = Add(x=5.0, y=w470) -> (x+y=w465:dbl)
            n98 = call "GetCCDPerformanceInfo.vi"("RO Speed Mode"=w465) -> ("Gain"=w475:dbl, "Read Noise"=w474:dbl)
            n99 = Add(x=w463, y=9) -> (x+y=w481:i32)
            n100 = call <vilib>:"Set Busy.vi"() -> ("error out"=w477:errorcluster)  [unwired: 10 in, 1 out]
            n101 = Bundle By Name(cluster=w473, "Other Info..CCD Gain"=w475, "Other Info..CCD Read Noise"=w474) -> (w472:T4)
            n102 = call "Send Single TCP-IP Cmd 1.vi"("TCP/IP ID"=w482, "Function #"=u16 1042, "Camera ID"=u8 1, "Acq. Mode/Type/Frame Mode/RO Mode #"=w481, "Error In"=w477) -> ("Error Out"=w485:errorcluster)  [unwired: 7 in, 3 out]
            n103 = local write "CCD Readout Speed"(w479) -> ()
            n104 = call "SI Image Error Handler - Win 2.vi"("error in (no error)"=w485) -> ("error out"=w476:errorcluster)  [unwired: 4 in]
            n105 = call <vilib>:"Unset Busy.vi"("error in (no error)"=w476) -> ()  [unwired: 10 in, 1 out]
            n106 = local write "Current Status"("Changing CCD port readout mode..." ("Current Status")) -> ()
            n107 = local write "Script"(w472) -> ()
          }
          event "Calculate Offset": Value Change {
            w512 = 0.0 ("f")
            w513 = 1.0 ("t")
            n108 = event-data() -> ()  [unwired: 1 in, 1 out]
            n109 = call "GetTCSInfo.vi"() -> ("TCSInfo"=w497:T12)
            n110 = Unbundle By Name(w497) -> ("Mount Az"=w490:dbl, "Rotator Angle"=w496:dbl, "Mount El"=w495:dbl)
            n111 = global read "TCSLINK_global.vi" "Position Angle"() -> (w486:dbl)
            n112 = local read "CCD ROI"() -> (w502:cluster{i32, i32, i32, i32, i32, i32})
            n113 = Subtract(x=w496, y=w495) -> (x-y=w489:dbl)
            n114 = Divide(x=3.141592653589793, y=180.0) -> (x/y=w493:dbl)
            n115 = Compound Arithmetic op=ADD(w490, w489, 180.0 ("value")) -> ()  [unwired: 1 out]
            n116 = Unbundle(w502) -> (w501:i32, w500:i32)  [unwired: 4 out]
            n117 = Multiply(x=w486, y=w493) -> (x*y=w487:dbl)
            n118 = formula code="ew_o = x_o*cos(p)*b_x+y_o*sin(p)*b_y;\nns_o = -x_o*sin(p)*b_x+y_o*cos(p)*b_y;\new_s = x_s*cos(p)*b_x+y_s*sin(p)*b_y;\nns_s = -x_s*sin(p)*b_x+y_s*cos(p)*b_y;\new_move=((ew_o-ew_s)*0.146);\nns_move=((ns_o-ns_s)*0.146);"("x_o"="ox1", "y_o"="oy1", "x_s"="sx1", "y_s"="sy1", "b_x"=w501, "b_y"=w500, "p"=w487) -> ("ew_move"=w509:dbl, "ns_move"=w510:dbl)  [unwired: 4 out]
            n119 = Less Than 0?(x=w510) -> (x < 0?=w514:bool)
            n120 = Select(t=w513, s=w514, f=w512) -> (s? t:f=w504:dbl)
            n121 = local write "N/S Offset Choice"(w504) -> ()
            n122 = Less Than 0?(x=w509) -> (x < 0?=w511:bool)
            n123 = Select(t=w513, s=w511, f=w512) -> (s? t:f=w503:dbl)
            n124 = local write "E/W Offset Choice"(w503) -> ()
            n125 = Absolute Value(x=w509) -> (abs(x)=w499:dbl)
            n126 = Absolute Value(x=w510) -> (abs(x)=w498:dbl)
            n127 = local write "E/W Offset"(w499) -> ()
            n128 = local write "N/S Offset"(w498) -> ()
            n129 = local write "Calculate Offset"(FALSE ("Calculate Offset")) -> ()
          }
          event "Lamp Cluster": Value Change {
            n130 = event-data() -> ("OldVal"=w518:T1, "NewVal"=w519:T1)  [unwired: 1 in]
            n131 = Cluster To Array(cluster=w519) -> (array=w520:bool[])
            n132 = Cluster To Array(cluster=w518) -> (array=w517:bool[])
            n133 = for {
              tunnel: w520 -> [w522] mode=indexing
              tunnel: w517 -> [w526] mode=indexing
              tunnel: w516 -> [w524]
              tunnel: w515 -> [w523]
              i -> [w525]
              n134 = Equal?(x=w526, y=w522) -> (x = y?=w521:bool)
              n135 = case shown="False" w521 {
                tunnel: w525 -> [_ w535]
                tunnel: w524 -> [_ w539]
                tunnel: w523 -> [_ w538]
                tunnel: w522 -> [_ w531]
                frame True {
                }
                frame False {
                  w533 = " " ("string")
                  n136 = property on="Lamp Cluster" class="Clust (strict)"() -> ("Controls[]"=w543:refnum<vi>[])  [unwired: 2 in, 2 out]
                  n137 = Index Array(array=w543, index=w535) -> (element=w534:refnum<vi>)
                  n138 = property class="Ctl"(reference=w534) -> ("Label.Text"=w542:string)  [unwired: 1 in, 2 out]
                  n139 = case shown="False" w531 {
                    tunnel: ["OFF" ("string") "ON" ("string")] -> w530
                    frame False {
                    }
                    frame True {
                    }
                  }
                  n140 = case shown="\"Ne\"" w542 {
                    tunnel: ["" "" "" "" w561 w563] -> w532
                    tunnel: ["L1" ("string") "L4" ("string") "L2" ("string") "L3" ("string") "L9" ("string") w563] -> w540
                    frame "Hg(Ar)" {
                    }
                    frame "Cu" {
                    }
                    frame "Ne" {
                    }
                    frame "Ar" {
                    }
                    frame "Quartz" {
                      n141 = Number To Decimal String(number="Quartz Intensity") -> (decimal integer string=w561:string)  [unwired: 1 in]
                    }
                    frame "", Default {
                      w563 = ""
                    }
                  }
                  n142 = Concatenate Strings("LAMP", w533, w540, w533, w530, w533, w532) -> (w529:string)
                  n143 = Enqueue Element(queue=w539, element=w529) -> ()  [unwired: 2 in, 3 out]
                  n144 = Dequeue Element(queue=w538, timeout in ms (-1)=2000) -> (element=w527:string)  [unwired: 1 in, 3 out]
                  n145 = Match Pattern(string=w527, regular expression="DONE") -> (offset past match=w536:i32)  [unwired: 1 in, 3 out]
                  n146 = case shown="-1" w536 {
                    tunnel: w534 -> [w551 _]
                    frame -1 {
                      n147 = property class="Ctl"(reference=w551) -> (reference out=w546:refnum<vi>, "Value"=w550:variant)  [unwired: 1 in, 1 out]
                      n148 = Variant To Data(type=TRUE, Variant=w550) -> (data=w549:bool)  [unwired: 1 in, 1 out]
                      n149 = Not(x=w549) -> (.not. x?=w548:bool)
                      n150 = property class="Ctl"(reference=w546, "Value"=w548) -> ()  [unwired: 1 in, 2 out]
                    }
                    frame 0, Default {
                    }
                  }
                }
              }
            }
          }
          event "Reset Wavelength Angles System": Value Change {
            n151 = event-data() -> ()  [unwired: 1 in, 6 out]
            n152 = Two Button Dialog(message="ARE YOU SURE you want to stop camera motion? ", 2:"YES" ("T button name (\"OK\")")) -> (T button?=w567:bool)  [unwired: 1 in]
            n153 = case shown="True" w567 {
              tunnel: w571 -> [w572 w577]
              tunnel: [w572 w576] -> w570
              tunnel: FALSE ("Reset Wavelength Angles System") -> [w573 w581]
              tunnel: [w573 w581] -> w565
              frame False {
              }
              frame True {
                n154 = Obtain Queue(name (unnamed)="WL_Command_Q", element data type=T5 {"Command"="", "Parameter"=""} ("Command"), error in (no error)=w577) -> (queue out=w575:refnum<queue>, error out=w580:errorcluster)  [unwired: 2 in, 1 out]
                n155 = Enqueue Element(queue=w575, element=T5 {"Command"="STOP_CAMERA_MOTION", "Parameter"=""}, error in (no error)=w580) -> (error out=w576:errorcluster)  [unwired: 1 in, 2 out]
              }
            }
            n156 = local write "Reset Wavelength Angles System"(w565) -> ()
            n157 = local write "Current Status"("Camera Rotation Stopped" ("Current Status")) -> ()
          }
          event "Start Exposure": Value Change {
            # "Gather information for FITS header file, change 'Exposure Acxtive?' to start image-taking sequence in 'POLL'"
            n158 = event-data() -> ()  [unwired: 1 in, 1 out]
            n159 = case shown="\"Object\"" "Exposure Tab" {
              tunnel: "Exp. Time (s)" -> [w610 w616 w622 w624 w630]
              tunnel: [w610 w616 w622 w624 w630] -> w594
              tunnel: ["# Dark Exposures" "# Zero Exposures" "# Exposures" "# Comp Exposures" "# Flat Exposures"] -> w593
              tunnel: ["Dark Comments:" "Zero Comments:" "Object Comments:" "Comp Comments:" "Flat Comments:"] -> w600
              tunnel: ["DARK" ("Object Name:") "ZERO" ("Object Name:") "Object Name:" "Comp Name:" "Flat Name:"] -> w601
              tunnel: [w606 w612 w618 w626 w634] -> w595
              tunnel: ["DARK" ("Other Info..OBSTYPE") "BIAS" ("Other Info..OBSTYPE") "OBJECT" ("Other Info..OBSTYPE") "COMP" ("Other Info..OBSTYPE") "FLAT" ("Other Info..OBSTYPE")] -> w586
              frame "Dark" {
                w606 = i16 0 items=["Dark", "Light"] ("Exposure type")
              }
              frame "Zero" {
                w612 = i16 0 items=["Dark", "Light"] ("Exposure type")
              }
              frame "Object" {
                w618 = i16 1 items=["Dark", "Light"] ("Exposure type")
              }
              frame "Comp" {
                w626 = i16 1 items=["Dark", "Light"] ("Exposure type")
              }
              frame "Flat" {
                w634 = i16 1 items=["Dark", "Light"] ("Exposure type")
              }
            }
            n160 = call "GetTCSInfo.vi"() -> ("TCSInfo"=w587:T12)
            n161 = Bundle By Name(cluster=T6 {"Object Name"="", "Telescope"="", "Instrument"="", "Comment"=""} ("input cluster"), "Object Name"=w601, "Telescope"="SOAR 4.1m", "Comment"=w600, "Instrument"="Goodman Spectrograph") -> (w597:T6)
            n162 = call "GetSystemsInfo.vi"() -> ("Pos Info"=w585:T13)
            n163 = call "GetComponentNames.vi"() -> ("Component Names"=w584:T14)
            n164 = Tick Count (ms)() -> (millisecond timer value=w589:u32)
            n165 = Bundle By Name(cluster=w591, "Obs parameters"=w597, "Current Exposure"=1, "Exposure type"=w595, "Exposure Active?"=TRUE, "#Exposures"=w593, "Exposure Time"=w594, "TCSInfo"=w587, "System Pos Info"=w585, "Component Names"=w584, "Last Exposure Start Time"=w589, "Other Info..OBSTYPE"=w586, "Other Info..OBSERVER"="Observer Name", "Other Info..Proposal #"="Proposal #") -> (w603:T4)
            n166 = local write "Script"(w603) -> ()
          }
          event "Show Images?": Value Change {
            n167 = event-data() -> ("NewVal"=w639:bool)  [unwired: 1 in]
            n168 = Current VI's Path() -> (path=w636:path)
            n169 = Strip Path(path=w636) -> (stripped path=w637:path)  [unwired: 1 out]
            n170 = Build Path(base path=w637, name or relative path="Quick_Look\\Quick_Look.vi") -> (appended path=w635:path)
            n171 = case shown="False" w639 {
              tunnel: w635 -> [_ w650]
              frame False {
                n172 = Obtain Queue(name (unnamed)="QUICKLOOK_Q", element data type=T5 {"Command"="", "Parameter"=""} ("element")) -> (queue out=w646:refnum<queue>, error out=w645:errorcluster)  [unwired: 3 in, 1 out]
                n173 = Enqueue Element(queue=w646, element=T5 {"Command"="SHUTDOWN", "Parameter"=""}, error in (no error)=w645) -> (queue out=w643:refnum<queue>, error out=w642:errorcluster)  [unwired: 1 in, 1 out]
                n174 = Release Queue(queue=w643, error in (no error)=w642) -> ()  [unwired: 1 in, 3 out]
              }
              frame True {
                n175 = Open VI Reference(vi path=w650) -> (vi reference=w651:refnum<vi>)  [unwired: 5 in, 1 out]
                n176 = invoke class="VI" method="FP.Open"(reference=w651) -> (reference out=w649:refnum<vi>)  [unwired: 4 in, 4 out]
                n177 = invoke class="VI" method="Run VI"(reference=w649, "Wait until done"=FALSE) -> (reference out=w647:refnum<vi>)  [unwired: 3 in, 4 out]
                n178 = Close Reference(reference=w647) -> ()  [unwired: 1 in, 1 out]
              }
            }
          }
          event "Take Thumbnail": Value Change {
            w666 = u16 1 items=["Retrieve Image Buffer", "Acquire and transfer to client", "Acquire and hold in Server Image Buffer", "Acquire, transfer to client, and save to Server's disk", "Acquire, save to Server's disk, and hold in Server Image Buffer"] ("Mode")
            w655 = 1 ("Current Exposure")
            # "Transfer instead of save"
            n179 = event-data() -> ()  [unwired: 1 in, 1 out]
            n180 = case shown="\"Check Star Focus\"" "Thumbnail Setting" {
              tunnel: [w678 w684] -> w660
              frame "Check Entire CCD", Default {
                w677 = 32 ("element")
                # "Take current ROI, bin by 4"
                n181 = local read "Port Readout"() -> (w671:u16)
                n182 = Greater Than 0?(x=w671) -> (x > 0?=w672:bool)
                n183 = Select(t=128 ("element"), s=w672, f=64 ("element")) -> (s? t:f=w670:i32)
                n184 = Bundle("element"=16, "element"=w670, "element"=w677, "element"=0, "element"=w670, "element"=w677) -> (w678:T15)  [unwired: 1 in]
              }
              frame "Check Star Focus" {
                w679 = 1 ("element")
                n185 = Bundle("element"=1964, "element"=200, "element"=w679, "element"=1948, "element"=200, "element"=w679) -> (w684:T15)  [unwired: 1 in]
              }
            }
            n186 = local read "Exposure Tab"() -> (w654:enum32{"Object", "Flat", "Comp", "Dark", "Zero"})
            n187 = case shown="\"Object\", Default" w654 {
              tunnel: [w667 w668 w669] -> w653
              frame "Object", Default {
                w667 = i16 1 items=["Dark", "Light"] ("Exposure type")
              }
              frame "Zero" {
                w668 = i16 0 items=["Dark", "Light"] ("Exposure type")
              }
              frame "Dark" {
                w669 = i16 0 items=["Dark", "Light"] ("Exposure type")
              }
            }
            n188 = property on="Mode" class="Ring (strict)"("Value"=w666) -> ()  [unwired: 2 in, 2 out]
            n189 = local read "Exp. Time (s)"() -> (w652:dbl)
            n190 = local write "Current Status"("Acquiring thumbnail of CCD image..." ("Current Status")) -> ()
            n191 = Bundle By Name(cluster=w658, "Exposure Active?"=TRUE, "Current Exposure"=w655, "#Exposures"=w655, "Exposure type"=w653, "Exposure Time"=w652) -> (w656:T4)
            n192 = local write "Script"(w656) -> ()
            n193 = call "Send Single TCP-IP Cmd 1.vi"("TCP/IP ID"=w659, "Function #"=u16 1043, "Camera ID"=u8 1, "CCD Format Parameters"=w660) -> ("Error Out"=w664:errorcluster)  [unwired: 8 in, 3 out]
            n194 = call "SI Image Error Handler - Win 2.vi"("error in (no error)"=w664) -> ()  [unwired: 4 in, 1 out]
          }
          event "MOS": Value Change {
            n195 = event-data() -> ("NewVal"=w685:bool)  [unwired: 1 in]
            n196 = Current VI's Path() -> (path=w687:path)
            n197 = Strip Path(path=w687) -> (stripped path=w688:path)  [unwired: 1 out]
            n198 = Build Path(base path=w688, name or relative path="Quick_Look\\MultiSlit_Graphical.vi") -> (appended path=w686:path)
            n199 = case shown="True" w685 {
              tunnel: w686 -> [_ w700]
              frame False {
                n200 = Obtain Queue(name (unnamed)="MULTISLIT_Q", element data type=T5 {"Command"="", "Parameter"=""} ("element")) -> (queue out=w696:refnum<queue>, error out=w695:errorcluster)  [unwired: 3 in, 1 out]
                n201 = Enqueue Element(queue=w696, element=T5 {"Command"="SHUTDOWN", "Parameter"=""}, error in (no error)=w695) -> (queue out=w693:refnum<queue>, error out=w692:errorcluster)  [unwired: 1 in, 1 out]
                n202 = Release Queue(queue=w693, error in (no error)=w692) -> ()  [unwired: 1 in, 3 out]
              }
              frame True {
                n203 = Open VI Reference(vi path=w700) -> (vi reference=w701:refnum<vi>)  [unwired: 5 in, 1 out]
                n204 = invoke class="VI" method="FP.Open"(reference=w701) -> (reference out=w699:refnum<vi>)  [unwired: 4 in, 4 out]
                n205 = invoke class="VI" method="Run VI"(reference=w699, "Wait until done"=FALSE) -> (reference out=w697:refnum<vi>)  [unwired: 3 in, 4 out]
                n206 = Close Reference(reference=w697) -> ()  [unwired: 1 in, 1 out]
              }
            }
          }
          event "Observer Name": Value Change {
            n207 = event-data() -> ()  [unwired: 1 in, 6 out]
            n208 = local read "Observer Name"() -> (w706:string)
            n209 = Search and Replace String(input string=w706, search string="'") -> (offset past replacement=w704:i32)  [unwired: 6 in, 3 out]
            n210 = Equal?(x=w704, y=-1) -> (x = y?=w702:bool)
            n211 = case shown="False" w702 {
              frame False {
                n212 = call "Display Message to User"() -> ()  [unwired: 10 in, 2 out]
              }
              frame True {
              }
            }
          }
          event "Offset Telescope": Value Change {
            w717 = " " ("string")
            w722 = "%1.2f" ("format string")
            w727 = 1 ("length (rest)")
            # "Send offset command to TCS, obtain response from TCS"
            n213 = event-data() -> ()  [unwired: 1 in, 1 out]
            n214 = property on="E/W Offset Choice" class="Ring (strict)"() -> ("Ring Text.Text"=w725:string)  [unwired: 2 in, 2 out]
            n215 = property on="N/S Offset Choice" class="Ring (strict)"() -> ("Ring Text.Text"=w726:string)  [unwired: 2 in, 2 out]
            n216 = Format Value(format string=w722, value (0)="E/W Offset") -> (output string=w719:string)  [unwired: 1 in]
            n217 = Format Value(format string=w722, value (0)="N/S Offset") -> (output string=w716:string)  [unwired: 1 in]
            n218 = String Subset(string=w725, length (rest)=w727) -> (substring=w723:string)  [unwired: 1 in]
            n219 = String Subset(string=w726, length (rest)=w727) -> (substring=w718:string)  [unwired: 1 in]
            n220 = Concatenate Strings("OFFSET MOVE ", w723, w717, w719, w717, w718, w717, w716) -> (w711:string)
            n221 = Enqueue Element(queue=w713, element=w711) -> (error out=w715:errorcluster)  [unwired: 2 in, 2 out]
            n222 = Dequeue Element(queue=w712, timeout in ms (-1)=2000, error in (no error)=w715) -> (element=w709:string)  [unwired: 3 out]
            n223 = Concatenate Strings("TCS: " ("string"), w709) -> (w708:string)
            n224 = flat-sequence {
              tunnel: w708 -> [_]
              tunnel: ["Applying SOAR offset..."] -> w707
              frame #0 {
                w729 = 0.0 ("E/W Offset")
                n225 = local write "Offset Telescope"(FALSE ("Offset Telescope")) -> ()
                n226 = local write "E/W Offset"(w729) -> ()
                n227 = local write "N/S Offset"(w729) -> ()
              }
            }
            n228 = local write "Current Status"(w707) -> ()
          }
          event "Reset TCP": Value Change {
            w732 = u8 0 ("Disabled")
            n229 = event-data() -> ()  [unwired: 1 in, 1 out]
            n230 = Enqueue Element(queue=w739, element=T5 {"Command"="INIT_TCP", "Parameter"=""}, error in (no error)=w738) -> (error out=w735:errorcluster)  [unwired: 1 in, 2 out]
            n231 = TCP Close Connection(connection ID=w740, error in (no error)=w735) -> (error out=w734:errorcluster)  [unwired: 1 in, 1 out]
            n232 = local write "Connection Status"(FALSE ("Connection Status")) -> ()
            n233 = local write "Reset TCP"(FALSE ("Reset TCP")) -> ()
            n234 = property on="Server Address" class="Str"("Disabled"=w732) -> ()  [unwired: 2 in, 2 out]
            n235 = property on="Port" class="DigNum (strict)"("Disabled"=w732) -> ()  [unwired: 2 in, 2 out]
            n236 = local write "Current Status"("Resetting TCP/IP connection..." ("Current Status")) -> ()
          }
          event "SHUTDOWN": Value Change {
            n237 = event-data() -> ()  [unwired: 1 in, 1 out]
            n238 = Enqueue Element(queue=w744, element=T5 {"Command"="SHUTDOWN", "Parameter"=""}, error in (no error)=w743) -> (error out=w742:errorcluster)  [unwired: 1 in, 2 out]
          }
        }
      }
      frame "ACCEPT_OFFSET_COORD" {
        w747 = 0.0 ("sx1")
        w745 = "%.1f" ("format string")
        w751 = " " ("regular expression")
        n239 = Match Pattern(string=w755, regular expression=w751) -> (before substring=w753:string, after substring=w754:string)  [unwired: 1 in, 2 out]
        n240 = Match Pattern(string=w754, regular expression=w751) -> (before substring=w750:string, after substring=w748:string)  [unwired: 1 in, 2 out]
        n241 = Scan Value(string=w750, format string=w745, default (0 dbl)=w747) -> (value=w749:dbl)  [unwired: 1 out]
        n242 = Scan Value(string=w748, format string=w745, default (0 dbl)=w747) -> (value=w746:dbl)  [unwired: 1 out]
        n243 = case shown="\"O\"" w753 {
          tunnel: w749 -> [w756 _ w759]
          tunnel: w746 -> [w757 _ w758]
          frame "O" {
            n244 = local write "ox1"(w756) -> ()
            n245 = local write "oy1"(w757) -> ()
          }
          frame Default {
          }
          frame "T" {
            n246 = local write "sx1"(w759) -> ()
            n247 = local write "sy1"(w758) -> ()
          }
        }
      }
      frame "INIT_TCP" {
        # "Establish TCP/ID connection with camera server; try again until connection sucessful."
        n248 = TCP Open Connection(address=w768, remote port or service name=w769, error in (no error)=w767) -> (connection ID=→"TCP/IP ID":refnum<k5>, error out=w763:errorcluster)  [unwired: 2 in]
        n249 = Unbundle By Name(w763) -> ("status"=w761:bool)
        n250 = case shown="True" w761 {
          tunnel: w764 -> [w773 w778]
          tunnel: ["TCP/IP connection established..." ("Current Status") "Trying to establish TCP/IP connection..." ("Current Status")] -> w760
          frame False {
            w775 = u8 1 ("Disabled")
            n251 = Enqueue Element(queue=w773, element=T5 {"Command"="INIT_CAMERA", "Parameter"=""}) -> (queue out=w771:refnum<queue>)  [unwired: 2 in, 2 out]
            n252 = Enqueue Element(queue=w771, element=T5 {"Command"="ENABLE_CONTROLS", "Parameter"=""}) -> ()  [unwired: 2 in, 3 out]
            n253 = property on="Server Address" class="Str"("Disabled"=w775) -> ()  [unwired: 2 in, 2 out]
            n254 = property on="Port" class="DigNum (strict)"("Disabled"=w775) -> ()  [unwired: 2 in, 2 out]
          }
          frame True {
            n255 = Enqueue Element(queue=w778, element=T5 {"Command"="INIT_TCP", "Parameter"=""}) -> ()  [unwired: 2 in, 3 out]
          }
        }
        n256 = Not(x=w761) -> (.not. x?=→"Connection Status":bool)
        n257 = local write "Current Status"(w760) -> ()
      }
      frame "INIT_CAMERA" {
        w786 = u16 2 items=["4-port", "Port A", "Port B", "Port C", "Port D"] ("Port Readout")
        w801 = u8 5 items=["50 kHz, ATTN 0", "50 kHz, ATTN 2", "50 kHz, ATTN 3", "100 kHz, ATTN 0", "100 kHz, ATTN 2", "100 kHz, ATTN 3", "200 kHz, ATTN 0", "200 kHz, ATTN 2", "400 kHz, ATTN 0"] ("CCD Readout Speed")
        w802 = u16 9 items=["Imaging, 1x1  ", "Imaging, 2x2", "Spectroscopic, 1x1", "Spectroscopic, 2x2", "Focus (Imag.)", "Focus (Spect.)", "Slicer", "Slit Imaging/Alignment", "Set user-defined ROI...", "Custom Mode"] ("CCD ROI Mode")
        # "Upon startup, set acquisition mode to \"Triggered Acquisition\""
        # "Upon startup, set tab to \"object\" , set exp time to 1sec."
        # "=100kHz ATTN3\non Port B"
        # "=100kHz ATTN3"
        # "Upon startup, set to Port B; proper gain and RDnoise for Port B, 100 kHz  ATTN 3 are default values in script"
        n258 = invoke on="Script" class="Clust (strict)" method="Reinit To Default"(error in=w800) -> (error out=w799:errorcluster)  [unwired: 2 in, 2 out]
        n259 = local read "CCD ROI"() -> (w798:cluster{i32, i32, i32, i32, i32, i32})
        n260 = local write "Port Readout"(w786) -> ()
        n261 = local write "CCD ROI Mode"(w802) -> ()
        n262 = local write "CCD Readout Speed"(w801) -> ()
        n263 = property on="Port Readout" class="Ring (strict)"("Visible"=FALSE) -> ()  [unwired: 2 in, 2 out]
        n264 = call "CalculateCCDReadoutTime.vi"("Readout Speed"=u8 5 ("Acq. Mode/Type/Frame Mode/RO Mode #"), "CCD ROI"=w798) -> ("Readout Time"=w797:dbl)
        n265 = call "Send Single TCP-IP Cmd 1.vi"("TCP/IP ID"=w804, "Function #"=u16 1042, "Camera ID"=u8 1, "Acq. Mode/Type/Frame Mode/RO Mode #"=u8 11, "Error In"=w799) -> ("TCP/IP ID Out"=w789:refnum<k5>, "Error Out"=w790:errorcluster)  [unwired: 7 in, 2 out]
        n266 = local write "Readout Time"(w797) -> ()
        n267 = local write "Exp. Time (s)"(1.0 ("Exp. Time (s)")) -> ()
        n268 = call "Send Single TCP-IP Cmd 1.vi"("TCP/IP ID"=w789, "Function #"=u16 1035, "Camera ID"=u8 1, "Exposure Time (ms)"=u32 1000, "Error In"=w790) -> ("TCP/IP ID Out"=w779:refnum<k5>, "Error Out"=w793:errorcluster)  [unwired: 7 in, 2 out]
        n269 = local write "Exposure Tab"(enum32{"Object", "Flat", "Comp", "Dark", "Zero"}."Object" ("Exposure Tab")) -> ()
        n270 = call "SI Image Error Handler - Win 2.vi"("error in (no error)"=w793) -> ("error out"=w782:errorcluster)  [unwired: 4 in]
        n271 = call "Send Single TCP-IP Cmd 1.vi"("TCP/IP ID"=w779, "Function #"=u16 1036, "Camera ID"=u8 1, "Acq. Mode/Type/Frame Mode/RO Mode #"=3, "Error In"=w782) -> ("Error Out"=w785:errorcluster)  [unwired: 7 in, 3 out]
        n272 = call "SI Image Error Handler - Win 2.vi"("error in (no error)"=w785) -> ("error out"=w781:errorcluster)  [unwired: 4 in]
      }
      frame "POLL" {
        # "Govern the image-taking sequence properly"
        n273 = Unbundle By Name(w815) -> ("Exposure Active?"=w816:bool)
        n274 = local read "Current Status"() -> (w809:string)
        n275 = case shown="True" w816 {
          tunnel: w815 -> [_ w842]
          tunnel: w814 -> [_ w841]
          tunnel: w812 -> [w829 w840]
          tunnel: [w827 w839] -> w813
          tunnel: w811 -> [w828 w838]
          frame False {
            n276 = case shown="True" "Get Camera Status" {
              tunnel: w829 -> [w830 w835]
              tunnel: w828 -> [_ w834]
              tunnel: [w830 w833] -> w827
              frame False {
              }
              frame True {
                n277 = call "GetCameraStatus.vi"("TCP/IP ID"=w834, "error in (no error)"=w835) -> ("CCD Temp."=→"CCD Temp.":sgl, "Vacuum Pressure"=→"Vacuum Pressure":sgl, "error out"=w833:errorcluster)  [unwired: 1 in, 1 out]
                n278 = property on="Get Camera Status" class="Bool (strict)"("Value"=FALSE ("Get Camera Status")) -> ()  [unwired: 2 in, 2 out]
                n279 = local write "Current Status"("Getting camera status..." ("Current Status")) -> ()
              }
            }
          }
          frame True {
            n280 = global read "Apogee_Global.vi" "Camera State"() -> (w843:T7)
            n281 = case shown="\"Ready\", Default" w843 {
              tunnel: w842 -> [_ w849]
              tunnel: w841 -> [w845 w852]
              tunnel: w840 -> [w846 w851]
              tunnel: [w847 w850] -> w839
              tunnel: w838 -> [_ _]
              frame "Exposing" {
                n282 = Enqueue Element(queue=w845, element=T5 {"Command"="START_SCRIPT", "Parameter"=""}, error in (no error)=w846) -> (error out=w847:errorcluster)  [unwired: 1 in, 2 out]
              }
              frame "Ready", Default {
                n283 = Unbundle By Name(w849) -> ("Current Exposure"=w854:i32, "#Exposures"=w853:i32)
                n284 = Greater?(x=w854, y=w853) -> (0:w848:bool)
                n285 = case shown="False" w848 {
                  tunnel: w852 -> [w863 w896]
                  tunnel: w851 -> [w862 w894]
                  tunnel: [w861 w897] -> w850
                  tunnel: w849 -> [_ w900]
                  frame False {
                    n286 = local read "Take Thumbnail"() -> (w857:bool)
                    n287 = Not(x=w857) -> (.not. x?=w856:bool)
                    n288 = local read "Mode"() -> (w860:u16)
                    n289 = Greater?(x=w860, y=u16 0) -> (0:w858:bool)
                    n290 = And(x=w858, y=w856) -> (x .and. y?=w855:bool)
                    n291 = case shown="True" w855 {
                      tunnel: w863 -> [w869 w889]
                      tunnel: w862 -> [w865 w887]
                      tunnel: [w871 w891] -> w861
                      frame True {
                        n292 = flat-sequence {
                          tunnel: w865 -> [w874]
                          tunnel: [w873] -> w864
                          frame #0 {
                            n293 = global write "GPS_Driver_Global.vi" "RODone"(FALSE) -> ()
                          }
                          frame #1 {
                            n294 = local read "Open Shutter During Image?"() -> (w876:bool)
                            n295 = case shown="True" w876 {
                              tunnel: [w877 w882] -> w873
                              tunnel: w874 -> [w877 w879]
                              tunnel: path "C:/Documents and Settings/observer/Desktop/GSCS/Systems/SIcamera_Control/GPS_Drivers/ReadExEventFINAL.vi" -> [_ w884]
                              frame False {
                              }
                              frame True {
                                n296 = Open VI Reference(vi path=w884, error in (no error)=w879) -> (vi reference=w883:refnum<vi>, error out=w878:errorcluster)  [unwired: 4 in]
                                n297 = invoke class="VI" method="Run VI"(reference=w883, error in=w878, "Wait until done"=FALSE, "Auto Dispose Ref"=TRUE) -> (error out=w882:errorcluster)  [unwired: 1 in, 4 out]
                              }
                            }
                          }
                        }
                        n298 = Enqueue Element(queue=w869, element=T5 {"Command"="DISABLE_CONTROLS", "Parameter"=""}, error in (no error)=w864) -> (queue out=w868:refnum<queue>, error out=w867:errorcluster)  [unwired: 1 in, 1 out]
                        n299 = Enqueue Element(queue=w868, element=T5 {"Command"="WRITE_FITS_HEADER", "Parameter"=""}, error in (no error)=w867) -> (error out=w871:errorcluster)  [unwired: 1 in, 2 out]
                      }
                      frame False {
                        n300 = Enqueue Element(queue=w889, element=T5 {"Command"="DISABLE_CONTROLS", "Parameter"=""}, error in (no error)=w887) -> (queue out=w888:refnum<queue>, error out=w886:errorcluster)  [unwired: 1 in, 1 out]
                        n301 = Enqueue Element(queue=w888, element=T5 {"Command"="START_SCRIPT", "Parameter"=""}, error in (no error)=w886) -> (error out=w891:errorcluster)  [unwired: 1 in, 2 out]
                      }
                    }
                  }
                  frame True {
                    n302 = Bundle By Name(cluster=w900, "Exposure Active?"=FALSE) -> (w899:T4)
                    n303 = Enqueue Element(queue=w896, element=T5 {"Command"="ENABLE_CONTROLS", "Parameter"=""}, error in (no error)=w894) -> (queue out=w895:refnum<queue>, error out=w893:errorcluster)  [unwired: 1 in, 1 out]
                    n304 = local write "Script"(w899) -> ()
                    n305 = Enqueue Element(queue=w895, element=T5 {"Command"="END_SCRIPT", "Parameter"=""}, error in (no error)=w893) -> (error out=w897:errorcluster)  [unwired: 1 in, 2 out]
                  }
                }
              }
            }
          }
        }
        n306 = case shown="\"Getting camera status...\"" w809 {
          selector: w809 -> [w819 _ _ _ _ _ _]
          tunnel: [w819 "DONE: SOAR offset applied" ("Current Status") "DONE: Camera status updated" ("Current Status") "DONE: CCD readout speed changed" ("Current Status") "DONE: Waiting for next command" ("Current Status") "DONE:  New ROI mode set" ("Current Status") "DONE: CCD port readout mode set" ("Current Status")] -> w810
          frame "", Default {
          }
          frame "Applying SOAR offset..." {
          }
          frame "Getting camera status..." {
          }
          frame "Changing CCD readout speed..." {
          }
          frame "Finalizing acquisition..." {
          }
          frame "Setting new ROI mode..." {
          }
          frame "Changing CCD port readout mode..." {
          }
        }
        n307 = local write "Current Status"(w810) -> ()
        n308 = global read "GSP_GUI_global.vi" "User Type"() -> (w808:i8)
        n309 = case shown="2, 3" w808 {
          tunnel: [FALSE ("Visible") TRUE ("Visible")] -> w807
          frame 0, Default {
          }
          frame 2, 3 {
          }
        }
        n310 = property on="Port Readout" class="Ring (strict)"("Visible"=w807) -> ()  [unwired: 2 in, 2 out]
        n311 = property on="Save As" class="Ring (strict)"("Visible"=w807) -> ()  [unwired: 2 in, 2 out]
      }
      frame "TAKE_IMAGE" {
        # "Code from SI camera client software..."
        n312 = Unbundle By Name(w904) -> ("Current Exposure"=w907:i32, "#Exposures"=w914:i32)
        n313 = Tick Count (ms)() -> (millisecond timer value=w905:u32)
        n314 = while {
          shift-right: [w940] -> _
          shift-left: TRUE -> [w941]
          shift-right: [w938] -> _
          shift-left: _ -> [w939]
          shift-right: [w936] -> _
          shift-left: 0 ("timeout ms (5000)") -> [w937]
          tunnel: w905 -> [w934]
          tunnel: w903 -> [w922]
          tunnel: w904 -> [w923]
          tunnel: w903 -> [w921]
          tunnel: w902 -> [w919]
          stop <- w942 continue-if-true
          # "This Wait was added to work with Linux"
          n315 = local read "Start Exposure"() -> (w924:bool)
          n316 = call "Parse TCP-IP Response 4.vi"("TCP/IP ID"=w922, "timeout ms (5000)"=100) -> ("Packet ID"=w944:u8, "Data Type"=w945:u16, "Command Done"=w950:cluster{"Function #":u16}, "Acq. Status"=w949:T16, "Image Packet"=w948:T17, "error out"=w947:errorcluster)  [unwired: 3 in, 5 out]
          n317 = case shown="No Error" w947 {
            selector: w947 -> [_ w1093]
            tunnel: w944 -> [w976 _]
            tunnel: w950 -> [w975 _]
            tunnel: w949 -> [w974 _]
            tunnel: [w973 w1094] -> w943
            tunnel: w945 -> [w972 _]
            tunnel: w939 -> [w971 w1096]
            tunnel: [w970 w1096] -> w938
            tunnel: [w969 w1091] -> w940
            tunnel: w948 -> [w968 _]
            tunnel: w941 -> [w967 w1091]
            tunnel: w937 -> [w966 w1092]
            tunnel: [w965 w1092] -> w936
            frame No Error {
              n318 = case shown="132" w976 {
                tunnel: w975 -> [_ _ _]
                tunnel: w974 -> [_ w987 _]
                tunnel: [TRUE w985 w1020] -> w973
                tunnel: w972 -> [_ w986 _]
                tunnel: w968 -> [_ _ w1033]
                tunnel: w971 -> [w979 w984 w1025]
                tunnel: [w979 w984 w1023] -> w970
                tunnel: [w978 w983 FALSE] -> w969
                tunnel: w967 -> [w978 w983 w1024]
                tunnel: w966 -> [w977 w982 w1022]
                tunnel: [w977 w982 w1021] -> w965
                frame 0, Default {
                  n319 = One Button Dialog(message="An unknown Packet Identifier was received.") -> ()  [unwired: 1 in, 1 out]
                }
                frame 131 {
                  n320 = case shown="2004" w986 {
                    tunnel: w987 -> [_ _ w1015]
                    tunnel: [TRUE FALSE TRUE] -> w985
                    frame 0, Default {
                    }
                    frame 2007 {
                      w989 = TRUE
                      # "Command Done"
                      n321 = local read "Image #"() -> (w990:i32)
                      n322 = local read "File Name Base"() -> (w994:string)
                      n323 = local read "Start Exposure"() -> (w991:bool)
                      n324 = case shown="True" w991 {
                        tunnel: [w1000 w1002] -> w992
                        tunnel: w990 -> [w1000 w1001]
                        frame False {
                        }
                        frame True {
                          n325 = Increment(x=w1001) -> (x+1=w1002:i32)
                          n326 = local write "Image #"(w1002) -> ()
                        }
                      }
                      n327 = Format Into String(format string="%04d", w992) -> (resulting string=w996:string)  [unwired: 2 in, 1 out]
                      n328 = Concatenate Strings(w996, "." ("string"), w994) -> (w993:string)
                      n329 = local write "Image File Name"(w993) -> ()
                      n330 = global write "Apogee_Global.vi" "Camera State"(CameraStates."Ready" ("Camera State")) -> ()
                      n331 = global write "GPS_Driver_Global.vi" "RODone"(w989) -> ()
                      n332 = local write "RO Done"(w989) -> ()
                    }
                    frame 2004 {
                      n333 = local read "% Complete"() -> (w1010:u16)
                      n334 = Unbundle By Name(w1015) -> ("% Exp."=w1005:u16, "%Readout"=w1008:u16)
                      n335 = Equal To 0?(x=w1008) -> (x = 0?=w1007:bool)
                      n336 = Greater?(x=w1010, y=w1008) -> (0:w1009:bool)
                      n337 = Less?(x=w1008, y=u16 100) -> (x < y?=w1013:bool)
                      n338 = Select(t=w1005, s=w1007, f=u16 100) -> (s? t:f=→"% Exposure":u16)
                      n339 = Not(x=w1013) -> (.not. x?=w1003:bool)
                      n340 = local write "RO Done"(w1003) -> ()
                      n341 = global write "GPS_Driver_Global.vi" "RODone"(w1003) -> ()
                      n342 = case shown="False" w1009 {
                        tunnel: [w1016 w1017] -> w1011
                        tunnel: w1008 -> [w1016 w1017]
                        frame False {
                        }
                        frame True {
                          n343 = local read "Acquiring"() -> (w1018:u32)
                          n344 = Increment(x=w1018) -> (x+1=w1019:u32)
                          n345 = local write "Acquiring"(w1019) -> ()
                        }
                      }
                      "% Complete" <- w1011
                    }
                  }
                }
                frame 132 {
                  n346 = Unbundle By Name(w1033) -> ("Image Data $"=w1035:string, "Image Type"=w1034:u16, "Serial Length"=w1032:u16, "Parallel Length"=w1031:u16, "Offset"=w1027:u32, "# of Packets"=w1030:u16)  [unwired: 1 out]
                  n347 = To Long Integer(number=w1031) -> (32bit integer=w1029:i32)
                  n348 = To Long Integer(number=w1032) -> (32bit integer=w1028:i32)
                  n349 = case shown="2" w1034 {
                    tunnel: [w1070 w1073 w1078 w1081 w1085 w1088] -> w1026
                    tunnel: w1035 -> [w1068 w1072 w1076 w1080 w1084 w1087]
                    frame 0, Default {
                      # "U16"
                      n350 = Type Cast(type=u16[] [] ("Array Constant"), x=w1068) -> (*(type *) &x=w1071:u16[])
                      n351 = To Single Precision Float(number=w1071) -> (single precision float=w1070:sgl[])
                    }
                    frame 1 {
                      # "I16"
                      n352 = Type Cast(type=i16[] [] ("Array Constant"), x=w1072) -> (*(type *) &x=w1075:i16[])
                      n353 = To Single Precision Float(number=w1075) -> (single precision float=w1073:sgl[])
                    }
                    frame 2 {
                      # "U32"
                      n354 = Type Cast(type=u32[] [] ("Array Constant"), x=w1076) -> (*(type *) &x=w1079:u32[])
                      n355 = To Single Precision Float(number=w1079) -> (single precision float=w1078:sgl[])
                    }
                    frame 3 {
                      # "I32"
                      n356 = Type Cast(type=i32[] [] ("Array Constant"), x=w1080) -> (*(type *) &x=w1083:i32[])
                      n357 = To Single Precision Float(number=w1083) -> (single precision float=w1081:sgl[])
                    }
                    frame 4 {
                      # "SGL"
                      n358 = Type Cast(type=sgl[] [] ("Array Constant"), x=w1084) -> (*(type *) &x=w1085:sgl[])
                    }
                    frame 5 {
                      # "DBL"
                      n359 = Type Cast(type=dbl[] [] ("Array Constant"), x=w1087) -> (*(type *) &x=w1090:dbl[])
                      n360 = To Single Precision Float(number=w1090) -> (single precision float=w1088:sgl[])
                    }
                  }
                  n361 = case shown="True" w1024 {
                    tunnel: w1025 -> [w1044 _]
                    tunnel: w1028 -> [_ w1056]
                    tunnel: w1029 -> [_ w1057]
                    tunnel: [w1045 w1066] -> w1023
                    tunnel: w1026 -> [w1052 w1065]
                    tunnel: w1022 -> [w1037 w1063]
                    tunnel: [w1042 w1055] -> w1021
                    tunnel: [w1051 w1062] -> w1020
                    tunnel: w1027 -> [w1043 w1060]
                    tunnel: w1030 -> [w1040 w1059]
                    frame False {
                      w1039 = 100.0 ("y")
                      n362 = Increment(x=w1037) -> (x+1=w1042:i32)
                      n363 = Less?(x=w1042, y=w1040) -> (x < y?=w1051:bool)
                      n364 = Divide(x=w1042, y=w1040) -> (x/y=w1047:dbl)
                      n365 = Divide(x=w1040, y=w1039) -> (x/y=w1041:dbl)
                      n366 = Multiply(x=w1047, y=w1039) -> (x*y=w1046:dbl)
                      n367 = To Unsigned Word Integer(number=w1041) -> (unsigned 16bit integer=w1038:u16)
                      n368 = Quotient & Remainder(x=w1042, y=w1038) -> (x-y*floor(x/y)=w1050:i32)  [unwired: 1 out]
                      n369 = To Unsigned Word Integer(number=w1046) -> (unsigned 16bit integer=w1048:u16)
                      n370 = Equal To 0?(x=w1050) -> (x = 0?=w1049:bool)
                      n371 = case shown="False" w1049 {
                        tunnel: w1048 -> [_ w1053]
                        frame False {
                        }
                        frame True {
                          n372 = local write "% Complete"(w1053) -> ()
                        }
                      }
                      n373 = Replace Array Subset(array=w1044, new element=w1052, index=w1043) -> (w1045:sgl[])
                    }
                    frame True {
                      w1054 = TRUE
                      n374 = Increment(x=w1063) -> (x+1=w1055:i32)
                      n375 = global write "GPS_Driver_Global.vi" "RODone"(w1054) -> ()
                      n376 = local write "RO Done"(w1054) -> ()
                      n377 = Less?(x=w1055, y=w1059) -> (x < y?=w1062:bool)
                      n378 = Multiply(x=w1056, y=w1057) -> (x*y=w1061:i32)
                      n379 = Initialize Array(sgl 0.0 ("Element Data"), w1061) -> (w1064:sgl[])
                      n380 = property on="% Complete" class="Slide (strict)"("Caption.Text"="%Transfered") -> ()  [unwired: 2 in, 2 out]
                      n381 = Replace Array Subset(array=w1064, new element=w1065, index=w1060) -> (w1066:sgl[])
                      "P Len" <- w1057
                      "S Len" <- w1056
                    }
                  }
                }
              }
            }
            frame Error {
              n382 = Unbundle By Name(w1093) -> ("code"=w1095:i32)
              n383 = case shown="0, Default" w1095 {
                tunnel: w1093 -> [w1100 _]
                tunnel: [w1098 TRUE] -> w1094
                frame 0, Default {
                  w1098 = FALSE
                  n384 = call <vilib>:"Simple Error Handler.vi"("error source (\" \")"="There was an error in a TCP/IP read during an Image Acquisition. ", "error in (no error)"=w1100) -> ("error out"=w1097:errorcluster)  [unwired: 3 in, 4 out]
                  n385 = local write "Error out"(w1097) -> ()
                  n386 = local write "Start Exposure"(w1098) -> ()
                }
                frame 56 {
                  # "Timeout -  Keep going"
                }
              }
            }
          }
          n387 = case shown="True" w924 {
            selector: w924 -> [_ w964]
            tunnel: [TRUE w964] -> w920
            tunnel: w923 -> [w963 _]
            tunnel: w921 -> [w954 _]
            tunnel: w919 -> [w952 _]
            frame False {
              n388 = Bundle By Name(cluster=w963, "#Exposures"=0) -> (w961:T4)
              n389 = local write "Script"(w961) -> ()
              n390 = call "Create Command Packet 3.vi"("Camera ID (1)"=u8 1 ("Camera ID"), "Buffer/Avg #/Frames"=u16 1 ("Buffer #"), "Function #"=u16 1018) -> ("Cmd Packet"=w956:string)  [unwired: 8 in]
              n391 = call "Flush TCP-IP Input Buffer.vi"("TCP/IP ID"=w954) -> ("TCP/IP ID Out"=w957:refnum<k5>)  [unwired: 4 in]
              n392 = call "Send TCP-IP Cmd and Get Ackn 3.vi"("TCP/IP ID In"=w957, "Cmd Packet"=w956) -> ("TCP/IP ID Out"=w953:refnum<k5>)  [unwired: 7 in, 6 out]
              n393 = call "Flush TCP-IP Input Buffer.vi"("TCP/IP ID"=w953) -> ()  [unwired: 4 in, 1 out]
              n394 = Enqueue Element(queue=w952, element=T5 {"Command"="ABORT_RECOVERY", "Parameter"=""}) -> ()  [unwired: 2 in, 3 out]
            }
            frame True {
            }
          }
          n395 = local read "Readout Time"() -> (w926:dbl)
          n396 = Multiply(x=w926, y=1000.0) -> (x*y=w925:dbl)
          n397 = local read "% Complete"() -> (w932:u16)
          n398 = local read "Exp. Time (s)"() -> (w928:dbl)
          n399 = local read "Mode"() -> (w933:u16)
          n400 = property on="% Complete" class="Slide (strict)"() -> ("Caption.Text"=w931:string)  [unwired: 2 in, 2 out]
          n401 = call "GetExposureStatus.vi"("Readout Time"=w925, "% Complete Caption"=w931, "Previous % Complete Value"=w932, "Exposure Time"=w928, "Mode #"=w933, "Initial Time"=w934) -> ("% Exposed"=w929:dbl, "% Complete"=w930:dbl)
          n402 = local write "% Complete"(w930) -> ()
          n403 = local write "% Exposure"(w929) -> ()
          n404 = And(x=w943, y=w920) -> (x .and. y?=w942:bool)
          n405 = Wait (ms)(milliseconds to wait=u32 0) -> ()  [unwired: 1 out]
        }
        n406 = Decrement(x=w907) -> (x-1=w906:i32)
        n407 = Number To Decimal String(number=w906) -> (decimal integer string=w912:string)  [unwired: 1 in]
        n408 = Number To Decimal String(number=w914) -> (decimal integer string=w910:string)  [unwired: 1 in]
        n409 = Concatenate Strings("Acquiring image " ("Current Status"), w912, " of " ("Current Status"), w910, " ... " ("Current Status")) -> (w908:string)
        n410 = local write "Current Status"(w908) -> ()
        n411 = global write "Apogee_Global.vi" "Camera State"(CameraStates."Ready" ("Camera State")) -> ()
      }
      frame "WRITE_FITS_HEADER" {
        # "Write FITS header file before taking image; change camera state to 'exposing', increase exposure # by 1"
        n412 = Unbundle By Name(w1138) -> ("Reduction Info."=w1111:T18, "Obs parameters"=w1134:T6, "System Pos Info"=w1121:T19, "Component Names"=w1119:T14, "Other Info."=w1127:T20)  [unwired: 2 out]
        n413 = Delete(path (use dialog)=path "C:/Program Files/SI Image SGL D/Other Parameters.txt" ("Path to FITS Header File"), error in=w1135) -> (deleted path=w1130:path, error out=w1131:errorcluster)  [unwired: 3 in, 1 out]
        n414 = call "WriteObsInfo.vi"("error in (no error)"=w1131, "Obs parameters"=w1134, "Path to FITS Header File"=w1130) -> ("error out"=w1133:errorcluster, "# of Entries (after)"=w1117:i16, "Path to FITS Header File"=w1132:path)  [unwired: 2 in]
        n415 = call "GetTCSInfo.vi"() -> ("TCSInfo"=w1109:T12)
        n416 = call "WriteTCSInfo.vi"("error in (no error)"=w1133, "# of Entries (before)"=w1117, "TCSInfo"=w1109, "Pathto FITS Header File"=w1132) -> ("error out"=w1118:errorcluster, "# of Entries (after)"=w1116:i16, "Path to FITS Header File"=w1120:path)  [unwired: 1 in]
        n417 = call "WriteGoodmanInfo.vi"("System Pos Info"=w1121, "error in (no error)"=w1118, "# of Entries (before)"=w1116, "Component Names"=w1119, "Path to FITS Header File"=w1120) -> ("error out"=w1112:errorcluster, "# of Entries (after)"=w1113:i16, "Path to FITS Header File"=w1115:path)  [unwired: 1 in]
        n418 = local read "Exp. Time (s)"() -> (w1128:dbl)
        n419 = Unbundle(w1127) -> ("CCD Read Noise"=w1126:dbl, "CCD Gain"=w1125:dbl, "OBSTYPE"=w1124:string, "OBSERVER"=w1123:string, "Proposal #"=w1122:string, "Equinox"=w1110:dbl)
        n420 = Bundle("Exp. Time (s)"=w1128, "CCD Read Noise"=w1126, "CCD Gain"=w1125, "OBSTYPE"=w1124, "OBSERVER"=w1123, "Proposal #"=w1122, "Equinox"=w1110) -> (w1114:T21)  [unwired: 1 in]
        n421 = local write "Current Status"("Writing FITS Header File...." ("Current Status")) -> ()
        n422 = global write "Apogee_Global.vi" "Camera State"(CameraStates."Exposing" ("Camera State")) -> ()
        n423 = call "WriteOtherInfo.vi"("error in (no error)"=w1112, "# of Entries (before)"=w1113, "Other Info"=w1114, "Path to FITS Header File"=w1115) -> ("error out"=w1106:errorcluster, "# of Entries (after)"=w1104:i16, "Path to FITS Header File"=w1108:path)  [unwired: 1 in]
        n424 = call "GetEnvironmentalInfo.vi"() -> ("Environmental Info"=w1102:T22)
        n425 = call "WriteEnvironmentInfo.vi"("error in (no error)"=w1106, "# of Entries (before)"=w1104, "EnvironmentalInfo"=w1102, "Pathto FITS Header File"=w1108) -> ("error out"=w1105:errorcluster, "# of Entries (after)"=w1103:i16, "Path to FITS Header File"=w1107:path)  [unwired: 1 in]
        n426 = call "WriteReductionInfo.vi"("error in (no error)"=w1105, "# of Entries (before)"=w1103, "Reduction Info."=w1111, "Path to FITS Header File"=w1107) -> ()  [unwired: 1 in, 3 out]
      }
      frame "DISABLE_CONTROLS" {
        w1142 = u8 1 ("Disabled")
        n427 = Enqueue Element(queue=w1141, element=T5 {"Command"="DISABLE", "Parameter"=""}) -> (queue out=w1140:refnum<queue>)  [unwired: 2 in, 2 out]
        n428 = Release Queue(queue=w1140) -> ()  [unwired: 2 in, 3 out]
        n429 = property on="Port Readout" class="Ring (strict)"("Disabled"=w1142) -> ()  [unwired: 2 in, 2 out]
        n430 = property on="CCD Readout Speed" class="Ring (strict)"("Disabled"=w1142) -> ()  [unwired: 2 in, 2 out]
        n431 = property on="Systems Status & Control" class="TabCtl (strict)"("Disabled"=w1142) -> ()  [unwired: 2 in, 2 out]
        n432 = local read "Take Thumbnail"() -> (w1146:bool)
        n433 = property on="File Name Base" class="Str"("Disabled"=w1142) -> ()  [unwired: 2 in, 2 out]
        n434 = property on="Save" class="Bool (strict)"("Disabled"=w1142) -> ()  [unwired: 2 in, 2 out]
        n435 = property on="Image #" class="DigNum (strict)"("Disabled"=w1142) -> ()  [unwired: 2 in, 2 out]
        n436 = Select(t=1.0, s=w1146, f=0.0) -> (s? t:f=w1143:dbl)
        n437 = property on="Exposure Tab" class="TabCtl (strict)"("Disabled"=w1142) -> ()  [unwired: 2 in, 2 out]
        n438 = property on="Thumbnail Setting" class="Enum (strict)"("Disabled"=w1142) -> ()  [unwired: 2 in, 2 out]
        n439 = property on="CCD ROI Mode" class="Ring (strict)"("Disabled"=w1142) -> ()  [unwired: 2 in, 2 out]
        n440 = property on="Take Thumbnail" class="Bool (strict)"("Disabled"=w1142) -> ()  [unwired: 2 in, 2 out]
        n441 = property on="Start Exposure" class="Bool (strict)"("Disabled"=w1143) -> ()  [unwired: 2 in, 2 out]
        n442 = property on="Get Camera Status" class="Bool (strict)"("Disabled"=w1142) -> ()  [unwired: 2 in, 2 out]
        n443 = property on="Save As" class="Ring (strict)"("Disabled"=w1142) -> ()  [unwired: 2 in, 2 out]
        n444 = property on="Acq Mode" class="Enum (strict)"("Disabled"=w1142) -> ()  [unwired: 2 in, 2 out]
        n445 = property on="Exp. Time (s)" class="DigNum (strict)"("Disabled"=w1142) -> ()  [unwired: 2 in, 2 out]
      }
      frame "START_SCRIPT" {
        # "Send acquisition command to camera"
        n446 = Unbundle By Name(w1155) -> ("Current Exposure"=w1158:i32)
        n447 = local read "Image #"() -> (w1154:i32)
        n448 = Increment(x=w1158) -> (x+1=w1157:i32)
        n449 = Format Into String(format string="%04d", w1154) -> (resulting string=w1152:string)  [unwired: 2 in, 1 out]
        n450 = Bundle By Name(cluster=w1155, "Current Exposure"=w1157) -> (w1156:T4)
        n451 = Concatenate Strings(w1152, "." ("string"), "File Name Base", ".fits" ("string")) -> (w1149:string)
        "Current File Name" <- w1149
        n452 = case shown="1..4, Default" "Mode" {
          selector: "Mode" -> [w1210 w1217]
          tunnel: [w1211 w1219] -> w1171
          tunnel: "Acq Mode" -> [_ w1215]
          tunnel: w1149 -> [_ w1214]
          frame 0 {
            n453 = call "Create Command Packet 3.vi"("Camera ID (1)"=u8 1 ("Camera ID"), "Mode"=w1210, "Buffer/Avg #/Frames"=u16 1 ("Buffer #"), "Function #"=u16 1019) -> ("Cmd Packet"=w1211:string)  [unwired: 7 in]
          }
          frame 1..4, Default {
            w1221 = u16 1037  # Function #
            w1218 = u32 1  # Buffer
            w1220 = u8 1  # Camera ID
            n454 = case shown="\"Single Image\", Default" w1215 {
              frame "Single Image", Default {
              }
              frame "Average Images" {
                n455 = local write "Acquiring"(u32 1 ("Acquiring")) -> ()
              }
            }
            n456 = call "Create Command Packet 3.vi"("Save As"="Save As", "File Name"=w1214, "Camera ID (1)"=w1220, "Mode"=w1217, "Buffer/Avg #/Frames"=w1218, "Function #"=w1221) -> ("Cmd Packet"=w1219:string)  [unwired: 5 in]
          }
        }
        n457 = local write "Script"(w1156) -> ()
        n458 = call "Flush TCP-IP Input Buffer.vi"("TCP/IP ID"=w1159) -> ("TCP/IP ID Out"=w1172:refnum<k5>)  [unwired: 4 in]
        n459 = call "Send TCP-IP Cmd and Get Ackn 3.vi"("TCP/IP ID In"=w1172, "Cmd Packet"=w1171) -> ("Accepted Flag"=w1161:bool, "error out"=w1170:errorcluster)  [unwired: 7 in, 5 out]
        n460 = Unbundle By Name(w1170) -> ("status"=w1164:bool)
        n461 = Not(x=w1164) -> (.not. x?=w1163:bool)
        n462 = Or(x=w1161, y=w1163) -> (x .or. y?=w1169:bool)
        n463 = case shown="True" w1169 {
          tunnel: w1168 -> [w1179 w1187]
          tunnel: w1162 -> [w1177 w1188]
          tunnel: [w1176 w1184] -> w1167
          frame False {
            n464 = Enqueue Element(queue=w1179, element=T5 {"Command"="START_SCRIPT", "Parameter"=""}, error in (no error)=w1177) -> (error out=w1176:errorcluster)  [unwired: 1 in, 2 out]
            n465 = One Button Dialog(message="The Command sent was not accepted by the Camera Server.") -> ()  [unwired: 1 in, 1 out]
          }
          frame True {
            n466 = Enqueue Element(queue=w1187, element=T5 {"Command"="TAKE_IMAGE", "Parameter"=""}, error in (no error)=w1188) -> (queue out=w1182:refnum<queue>, error out=w1183:errorcluster)  [unwired: 1 in, 1 out]
            n467 = local read "Open Shutter During Image?"() -> (w1185:bool)
            n468 = Enqueue Element(queue=w1182, element=T5 {"Command"="SEND_IMAGE", "Parameter"=""}, error in (no error)=w1183) -> (error out=w1180:errorcluster)  [unwired: 1 in, 2 out]
            n469 = case shown="True" w1185 {
              tunnel: w1180 -> [w1192 w1200]
              tunnel: [w1191 w1199] -> w1184
              frame False {
                n470 = Number To Decimal String(number=500) -> (decimal integer string=w1194:string)  [unwired: 1 in]
                n471 = Build Array(w1194) -> (w1195:string[])
                n472 = call "gsp_silvermax_commandreponse.vi"("error in (no error)"=w1192, "Parameters (none)"=w1195, "Motor #"=u8 40, "Command"=T8."LRP (156)") -> ("error out"=w1191:errorcluster)  [unwired: 3 out]
              }
              frame True {
                n473 = local read "Exp. Time (s)"() -> (w1197:dbl)
                n474 = Multiply(x=w1197, y=8333.33) -> (x*y=w1198:dbl)
                n475 = To Long Integer(number=w1198) -> (32bit integer=w1206:i32)
                n476 = call "gsp_silvermax_writeregister.vi"("Register Value"=w1206, "Motor #"=u8 40, "Register# (0)"=u8 5) -> ("Motor # dup"=w1204:u8)  [unwired: 3 in, 1 out]
                n477 = Number To Decimal String(number=450) -> (decimal integer string=w1203:string)  [unwired: 1 in]
                n478 = Build Array(w1203) -> (w1201:string[])
                n479 = call "gsp_silvermax_commandreponse.vi"("error in (no error)"=w1200, "Parameters (none)"=w1201, "Motor #"=w1204, "Command"=T8."LRP (156)") -> ("error out"=w1199:errorcluster)  [unwired: 3 out]
              }
            }
          }
        }
        n480 = local write "Current Status"("Initializing acquisition..." ("Current Status")) -> ()
        n481 = property on="% Complete" class="Slide (strict)"("Caption.Text"="% Readout") -> ()  [unwired: 2 in, 2 out]
        n482 = local write "RO Done"(FALSE ("RO Done")) -> ()
      }
      frame "ABORT_RECOVERY" {
        n483 = Multiply(x=0.5, y=8333.33) -> (x*y=w1227:dbl)
        n484 = To Long Integer(number=w1227) -> (32bit integer=w1233:i32)
        n485 = call "gsp_silvermax_writeregister.vi"("Register Value"=w1233, "Motor #"=u8 40, "Register# (0)"=u8 5) -> ("Motor # dup"=w1231:u8)  [unwired: 3 in, 1 out]
        n486 = Number To Decimal String(number=450) -> (decimal integer string=w1230:string)  [unwired: 1 in]
        n487 = Build Array(w1230) -> (w1228:string[])
        n488 = call "gsp_silvermax_commandreponse.vi"("error in (no error)"=w1225, "Parameters (none)"=w1228, "Motor #"=w1231, "Command"=T8."LRP (156)") -> ("error out"=w1224:errorcluster)  [unwired: 3 out]
      }
      frame "SEND_IMAGE" {
        n489 = case shown="True" "Show Images?" {
          frame False {
          }
          frame True {
            n490 = local read "Current File Name"() -> (w1238:string)
            n491 = Obtain Queue(name (unnamed)="QUICKLOOK_Q", element data type=T5 {"Command"="", "Parameter"=""} ("element")) -> (queue out=w1243:refnum<queue>)  [unwired: 3 in, 2 out]
            n492 = Bundle("Command"="OPEN_FITS_FILE", "Current File Name"=w1238) -> (w1240:T23)  [unwired: 1 in]
            n493 = Enqueue Element(queue=w1243, element=w1240) -> (queue out=w1239:refnum<queue>)  [unwired: 2 in, 2 out]
            n494 = Release Queue(queue=w1239) -> ()  [unwired: 2 in, 3 out]
          }
        }
      }
      frame "MULTISLIT" {
        n495 = case shown="True" "MOS" {
          frame False {
          }
          frame True {
            n496 = local read "Current File Name"() -> (w1247:string)
            n497 = Obtain Queue(name (unnamed)="MULTISLIT_Q", element data type=T5 {"Command"="", "Parameter"=""} ("element")) -> (queue out=w1252:refnum<queue>)  [unwired: 3 in, 2 out]
            n498 = Bundle("Command"="OPEN_FITS_FILE", "Current File Name"=w1247) -> (w1249:T23)  [unwired: 1 in]
            n499 = Enqueue Element(queue=w1252, element=w1249) -> (queue out=w1248:refnum<queue>)  [unwired: 2 in, 2 out]
            n500 = Release Queue(queue=w1248) -> ()  [unwired: 2 in, 3 out]
          }
        }
      }
      frame "END_SCRIPT" {
        # "Check for success of acquisition"
        n501 = property on="Take Thumbnail" class="Bool (strict)"() -> ("Value"=w1258:bool)  [unwired: 2 in, 2 out]
        n502 = local read "Mode"() -> (w1264:u16)
        n503 = local read "Acq Mode"() -> (w1265:T3)
        n504 = case shown="True" w1258 {
          tunnel: w1259 -> [w1267 w1272]
          tunnel: [w1267 w1272] -> w1256
          tunnel: w1255 -> [_ w1269]
          frame False {
          }
          frame True {
            n505 = local write "Mode"(4) -> ()
            n506 = local read "CCD ROI"() -> (w1268:cluster{i32, i32, i32, i32, i32, i32})
            n507 = property on="Take Thumbnail" class="Bool (strict)"("Value"=FALSE ("Take Thumbnail")) -> ()  [unwired: 2 in, 2 out]
            n508 = call "Send Single TCP-IP Cmd 1.vi"("TCP/IP ID"=w1269, "Function #"=u16 1043, "Camera ID"=u8 1, "CCD Format Parameters"=w1268) -> ("Error Out"=w1273:errorcluster)  [unwired: 8 in, 3 out]
            n509 = call "SI Image Error Handler - Win 2.vi"("error in (no error)"=w1273) -> ()  [unwired: 4 in, 1 out]
          }
        }
        n510 = property on="Start Exposure" class="Bool (strict)"(error in=w1256, "Value"=FALSE ("Start Exposure")) -> (error out=w1260:errorcluster)  [unwired: 1 in, 1 out]
        n511 = property on="% Complete" class="Slide (strict)"(error in=w1260, "Caption.Text"="% Readout") -> (error out=w1257:errorcluster)  [unwired: 1 in, 1 out]
        n512 = case shown="1, Default" w1264 {
          selector: w1264 -> [w1278 w1280 w1305]
          tunnel: w1255 -> [_ w1279 _]
          tunnel: [w1278 w1280 w1305] -> w1266
          tunnel: w1265 -> [_ w1285 _]
          tunnel: [w1277 w1282 w1304] -> w1254
          tunnel: w1257 -> [w1277 w1281 w1304]
          frame 0 {
          }
          frame 1, Default {
            # "If Exposure was not 100%, acquisition was terminated so send TerminateAcquisition command."
            n513 = Equal?(x=w1285, y=Client_Acquisition_Mode_Menu."Average Images") -> (x = y?=w1283:bool)
            n514 = local read "# to Average"() -> (w1289:u32)
            n515 = local read "% Exposure"() -> (w1292:u16)
            n516 = local read "Acquiring"() -> (w1290:u32)
            n517 = Less?(x=w1290, y=w1289) -> (x < y?=w1288:bool)
            n518 = Less?(x=w1292, y=u16 100) -> (x < y?=w1287:bool)
            n519 = Select(t=w1288, s=w1283, f=w1287) -> (s? t:f=w1286:bool)
            n520 = case shown="True" w1286 {
              tunnel: w1279 -> [_ w1302]
              tunnel: [w1293 w1294] -> w1282
              tunnel: w1281 -> [w1293 _]
              frame False {
              }
              frame True {
                n521 = call "Create Command Packet 3.vi"("Camera ID (1)"=u8 1 ("Camera ID"), "Function #"=u16 1018) -> ("Cmd Packet"=w1300:string)  [unwired: 9 in]
                n522 = call "Flush TCP-IP Input Buffer.vi"("TCP/IP ID"=w1302) -> ("TCP/IP ID Out"=w1296:refnum<k5>)  [unwired: 4 in]
                n523 = TCP Write(connection ID=w1296, data in=w1300) -> (error out=w1299:errorcluster)  [unwired: 2 in, 2 out]
                n524 = call "Parse TCP-IP Response 4.vi"("TCP/IP ID"=w1296, "error in (no error)"=w1299) -> ("Packet Error Code"=→"Packet\nError code":i32, "Command Done"=w1298:cluster{"Function #":u16}, "error out"=w1294:errorcluster)  [unwired: 3 in, 8 out]
                n525 = Unbundle By Name(w1298) -> ("Function #"=→"Function #":u16)
              }
            }
          }
          frame 5 {
          }
        }
        n526 = stacked-sequence {
          tunnel: w1266 -> [_]
          frame #0 {
            w1276 = u16 0 ("% Exposure")
            n527 = local write "% Exposure"(w1276) -> ()
            n528 = local write "% Complete"(w1276) -> ()
            "Acquiring" <- w1276
          }
        }
        n529 = local write "Current Status"("Finalizing acquisition..." ("Current Status")) -> ()
      }
      frame "ENABLE_CONTROLS" {
        w1309 = u8 0 ("Disabled")
        n530 = property on="Acq Mode" class="Enum (strict)"("Disabled"=w1309) -> ()  [unwired: 2 in, 2 out]
        n531 = property on="Save As" class="Ring (strict)"("Disabled"=w1309) -> ()  [unwired: 2 in, 2 out]
        n532 = property on="Image #" class="DigNum (strict)"("Disabled"=w1309) -> ()  [unwired: 2 in, 2 out]
        n533 = property on="Thumbnail Setting" class="Enum (strict)"("Disabled"=w1309) -> ()  [unwired: 2 in, 2 out]
        n534 = property on="Get Camera Status" class="Bool (strict)"("Disabled"=w1309) -> ()  [unwired: 2 in, 2 out]
        n535 = property on="Exp. Time (s)" class="DigNum (strict)"("Disabled"=w1309) -> ()  [unwired: 2 in, 2 out]
        n536 = property on="File Name Base" class="Str"("Disabled"=w1309) -> ()  [unwired: 2 in, 2 out]
        n537 = property on="Exposure Tab" class="TabCtl (strict)"("Disabled"=w1309) -> ()  [unwired: 2 in, 2 out]
        n538 = Enqueue Element(queue=w1308, element=T5 {"Command"="ENABLE", "Parameter"=""}) -> (queue out=w1307:refnum<queue>)  [unwired: 2 in, 2 out]
        n539 = Release Queue(queue=w1307) -> ()  [unwired: 2 in, 3 out]
        n540 = property on="Take Thumbnail" class="Bool (strict)"("Disabled"=w1309) -> ()  [unwired: 2 in, 2 out]
        n541 = property on="Start Exposure" class="Bool (strict)"("Disabled"=w1309) -> ()  [unwired: 2 in, 2 out]
        n542 = property on="CCD ROI Mode" class="Ring (strict)"("Disabled"=w1309) -> ()  [unwired: 2 in, 2 out]
        n543 = property on="Port Readout" class="Ring (strict)"("Disabled"=w1309) -> ()  [unwired: 2 in, 2 out]
        n544 = property on="CCD Readout Speed" class="Ring (strict)"("Disabled"=w1309) -> ()  [unwired: 2 in, 2 out]
        n545 = property on="Systems Status & Control" class="TabCtl (strict)"("Disabled"=w1309) -> ()  [unwired: 2 in, 2 out]
      }
      frame "ERROR" {
        n546 = local read "Camera Errors"() -> (w1318:errorcluster)
        n547 = Bundle By Name(cluster=T9 {"error in (no error)"={"status"=FALSE, "code"=0, "source"=""}, "Source"="", "Comment "=""} ("Log"), "error in (no error)"=w1318, "Source"="SIcamera Control Module") -> (w1315:T9)
        n548 = call "GSP_Logger_Handler.vi"("Log"=w1315, "Actions"=T10."Log") -> ()  [unwired: 5 in, 1 out]
        n549 = Unbundle By Name(w1318) -> ("code"=w1317:i32)
        n550 = case shown="0, Default" w1317 {
          tunnel: w1318 -> [_ w1327]
          tunnel: [errorcluster {"status"=FALSE, "code"=0, "source"=""} ("last_camera_error") w1327] -> w1319
          tunnel: w1312 -> [w1323 w1326]
          tunnel: [w1323 w1326] -> w1311
          frame 0, Default {
            n551 = global write "Apogee_Global.vi" "Camera State"(CameraStates."Error" ("Camera State")) -> ()
          }
          frame 56 {
          }
        }
        n552 = case shown="Error" w1319 {
          tunnel: w1311 -> [_ w1321]
          frame No Error {
          }
          frame Error {
            n553 = Enqueue Element At Opposite End(queue=w1321, element=T5 {"Command"="SHUTDOWN", "Parameter"=""}) -> ()  [unwired: 2 in, 3 out]
          }
        }
      }
      frame "SHUTDOWN" {
        w1345 = u8 0 ("Disabled")
        n554 = Release Queue(queue=w1342) -> ()  [unwired: 2 in, 3 out]
        n555 = Release Queue(queue=w1343) -> ()  [unwired: 2 in, 3 out]
        n556 = Release Queue(queue=w1351, error in (no error)=w1350) -> (error out=w1348:errorcluster)  [unwired: 1 in, 2 out]
        n557 = TCP Close Connection(connection ID=w1344, error in (no error)=w1348) -> (error out=w1347:errorcluster)  [unwired: 1 in, 1 out]
        n558 = Obtain Queue(name (unnamed)="MULTISLIT_Q", element data type=T5 {"Command"="", "Parameter"=""} ("element")) -> (queue out=w1334:refnum<queue>, error out=w1333:errorcluster)  [unwired: 3 in, 1 out]
        n559 = Obtain Queue(name (unnamed)="QUICKLOOK_Q", element data type=T5 {"Command"="", "Parameter"=""} ("element")) -> (queue out=w1341:refnum<queue>, error out=w1340:errorcluster)  [unwired: 3 in, 1 out]
        n560 = Enqueue Element(queue=w1334, element=T5 {"Command"="SHUTDOWN", "Parameter"=""}, error in (no error)=w1333) -> (queue out=w1331:refnum<queue>, error out=w1330:errorcluster)  [unwired: 1 in, 1 out]
        n561 = Enqueue Element(queue=w1341, element=T5 {"Command"="SHUTDOWN", "Parameter"=""}, error in (no error)=w1340) -> (queue out=w1338:refnum<queue>, error out=w1337:errorcluster)  [unwired: 1 in, 1 out]
        n562 = Release Queue(queue=w1331, error in (no error)=w1330) -> ()  [unwired: 1 in, 3 out]
        n563 = Release Queue(queue=w1338, error in (no error)=w1337) -> ()  [unwired: 1 in, 3 out]
        n564 = property on="Server Address" class="Str"("Disabled"=w1345) -> ()  [unwired: 2 in, 2 out]
        n565 = property on="Port" class="DigNum (strict)"("Disabled"=w1345) -> ()  [unwired: 2 in, 2 out]
        n566 = local write "Connection Status"(FALSE ("Connection Status")) -> ()
        n567 = local write "Current Status"("Shutting down..." ("Current Status")) -> ()
      }
    }
    n568 = Equal?(x=w22, y="SHUTDOWN") -> (x = y?=w24:bool)
    n569 = case shown="No Error" w25 {
      selector: w25 -> [_ w35]
      tunnel: w26 -> [_ w37]
      frame No Error {
      }
      frame Error {
        n570 = Enqueue Element At Opposite End(queue=w37, element=T5 {"Command"="ERROR", "Parameter"=""}) -> ()  [unwired: 2 in, 3 out]
        "Camera Errors" <- w35
      }
    }
  }
